vi "tvac_gui_chamber.vi"() -> ()   [LabVIEW 2016]
uses:
  <vilib>/httpClient/LabVIEWHTTPClient.lvlib
  <vilib>/httpClient/ClientHandle.ctl
  msg7171_linux.llb/send single message.vi
  <vilib>/httpClient/POSTBuffer.vi
panel:
  in  "read pressure":bool
  out "headers":string
  in  "ThermalProfile":bool
  in  "Read Zones":bool
  out "value":cluster{"ZoneSetPoint":dbl[], "ZoneTemp":dbl[]}
  in  "Read MCC":bool
  out "output cluster":T1
  out "Cluster":T2
  in  "Custom Graph Selector":i32
  in  "exit":bool
  in  "AlarmColor":u32(colorbox)
  in  "Alarm String":string
  in  "Plot Color":u32(colorbox)=16860
  in  "Temperature":dbl format="%#_13g"
  in  "TC Label":string
  in  "Graph ON/OFF":u32(colorbox)=4250624
  in  "index (col)":i32
  in  "index (row)":i32
  out "working array":bool[](array[boolean])
  in  "Local Debug":bool
  in  "Tab Control":enum32{"TCs", "Graphs", "Thermal Profile"}(tab)
  in  "Log/Linear Y-Axis":u16(ring) items=["Linear", "Log"]
  in  "Total Time":dbl
  in  "Set Time TC Graph":bool
  in  "Graphing Selection":u16(ring) items=["User Selection", "Graph All Thermocouples", "Clear Graph"]
  in  "Time Scale":u16(ring) items=["Minutes", "Hours", "Seconds"]
  out "Waveform Chart":waveform(dbl)[](graph)
  out "Thermocouples":T3(array[cluster])
  in  "Log/Linear Y-Axis 6":u16(ring) items=["Linear", "Log"]
  in  "Log/Linear Y-Axis 5":u16(ring) items=["Linear", "Log"]
  in  "Log/Linear Y-Axis 3":u16(ring) items=["Linear", "Log"]
  in  "Log/Linear Y-Axis 2":u16(ring) items=["Linear", "Log"]
  in  "Total Time 6":dbl
  in  "Set Time TC Graph 6":bool
  in  "Time Scale 6":u16(ring) items=["Minutes", "Hours", "Seconds"]
  in  "Total Time 5":dbl
  in  "Set Time TC Graph 5":bool
  in  "Time Scale 5":u16(ring) items=["Minutes", "Hours", "Seconds"]
  in  "Total Time 4":dbl
  in  "Set Time TC Graph 4":bool
  in  "Time Scale 4":u16(ring) items=["Minutes", "Hours", "Seconds"]
  in  "Total Time 3":dbl
  in  "Set Time TC Graph 3":bool
  in  "Time Scale 3":u16(ring) items=["Minutes", "Hours", "Seconds"]
  in  "Total Time 2":dbl
  in  "Set Time TC Graph 2":bool
  in  "Time Scale 2":u16(ring) items=["Minutes", "Hours", "Seconds"]
  in  "Log/Linear Y-Axis 1":u16(ring) items=["Linear", "Log"]
  in  "Total Time 1":dbl
  in  "Set Time TC Graph 1":bool
  in  "Time Scale 1":u16(ring) items=["Minutes", "Hours", "Seconds"]
  in  "Custom Chart 2 Selection":i32[](listbox)=[0]
  in  "Custom Chart 1 Selection":i32[](listbox)=[0]
  out "Custom Chart 1":waveform(dbl)[](graph)
  in  "Custom Chart 3 Selection":i32[](listbox)=[0]
  in  "Custom Chart 4 Selection":i32[](listbox)=[0]
  in  "Custom Chart 5 Selection":i32[](listbox)=[0]
  in  "Custom Chart 6 Selection":i32[](listbox)=[0]
  out "Custom Chart 2":waveform(dbl)[](graph)
  out "Custom Chart 3":waveform(dbl)[](graph)
  out "Custom Chart 4":waveform(dbl)[](graph)
  out "Custom Chart 5":waveform(dbl)[](graph)
  out "Custom Chart 6":waveform(dbl)[](graph)
  in  "Log/Linear Y-Axis 4":u16(ring) items=["Linear", "Log"]
  in  "Run Profile 2":bool
  in  "Run Profile":bool
  in  "Resume Profile":bool
  in  "Stop Profile":bool
  in  "Pause Profile":bool
  in  "Hold Profile":bool
  in  "Set Z 1":bool
  in  "Z3 Thermal Profile":i32(listbox)
  in  "Z2 Thermal Profile":i32(listbox)
  in  "Z1 Thermal Profile":i32(listbox)
  in  "Zone 3 Temp":u16(ring) items=["Average", "Minimum", "Maximum"]
  in  "Zone 2 Temp":u16(ring) items=["Average", "Minimum", "Maximum"]
  in  "Zone 1 Temp":u16(ring) items=["Average", "Minimum", "Maximum"]
  in  "Zone 1 TC":i32[](listbox)=[0]
  in  "Zone 2 TC":i32[](listbox)=[0]
  in  "Zone 3 TC":i32[](listbox)=[0]
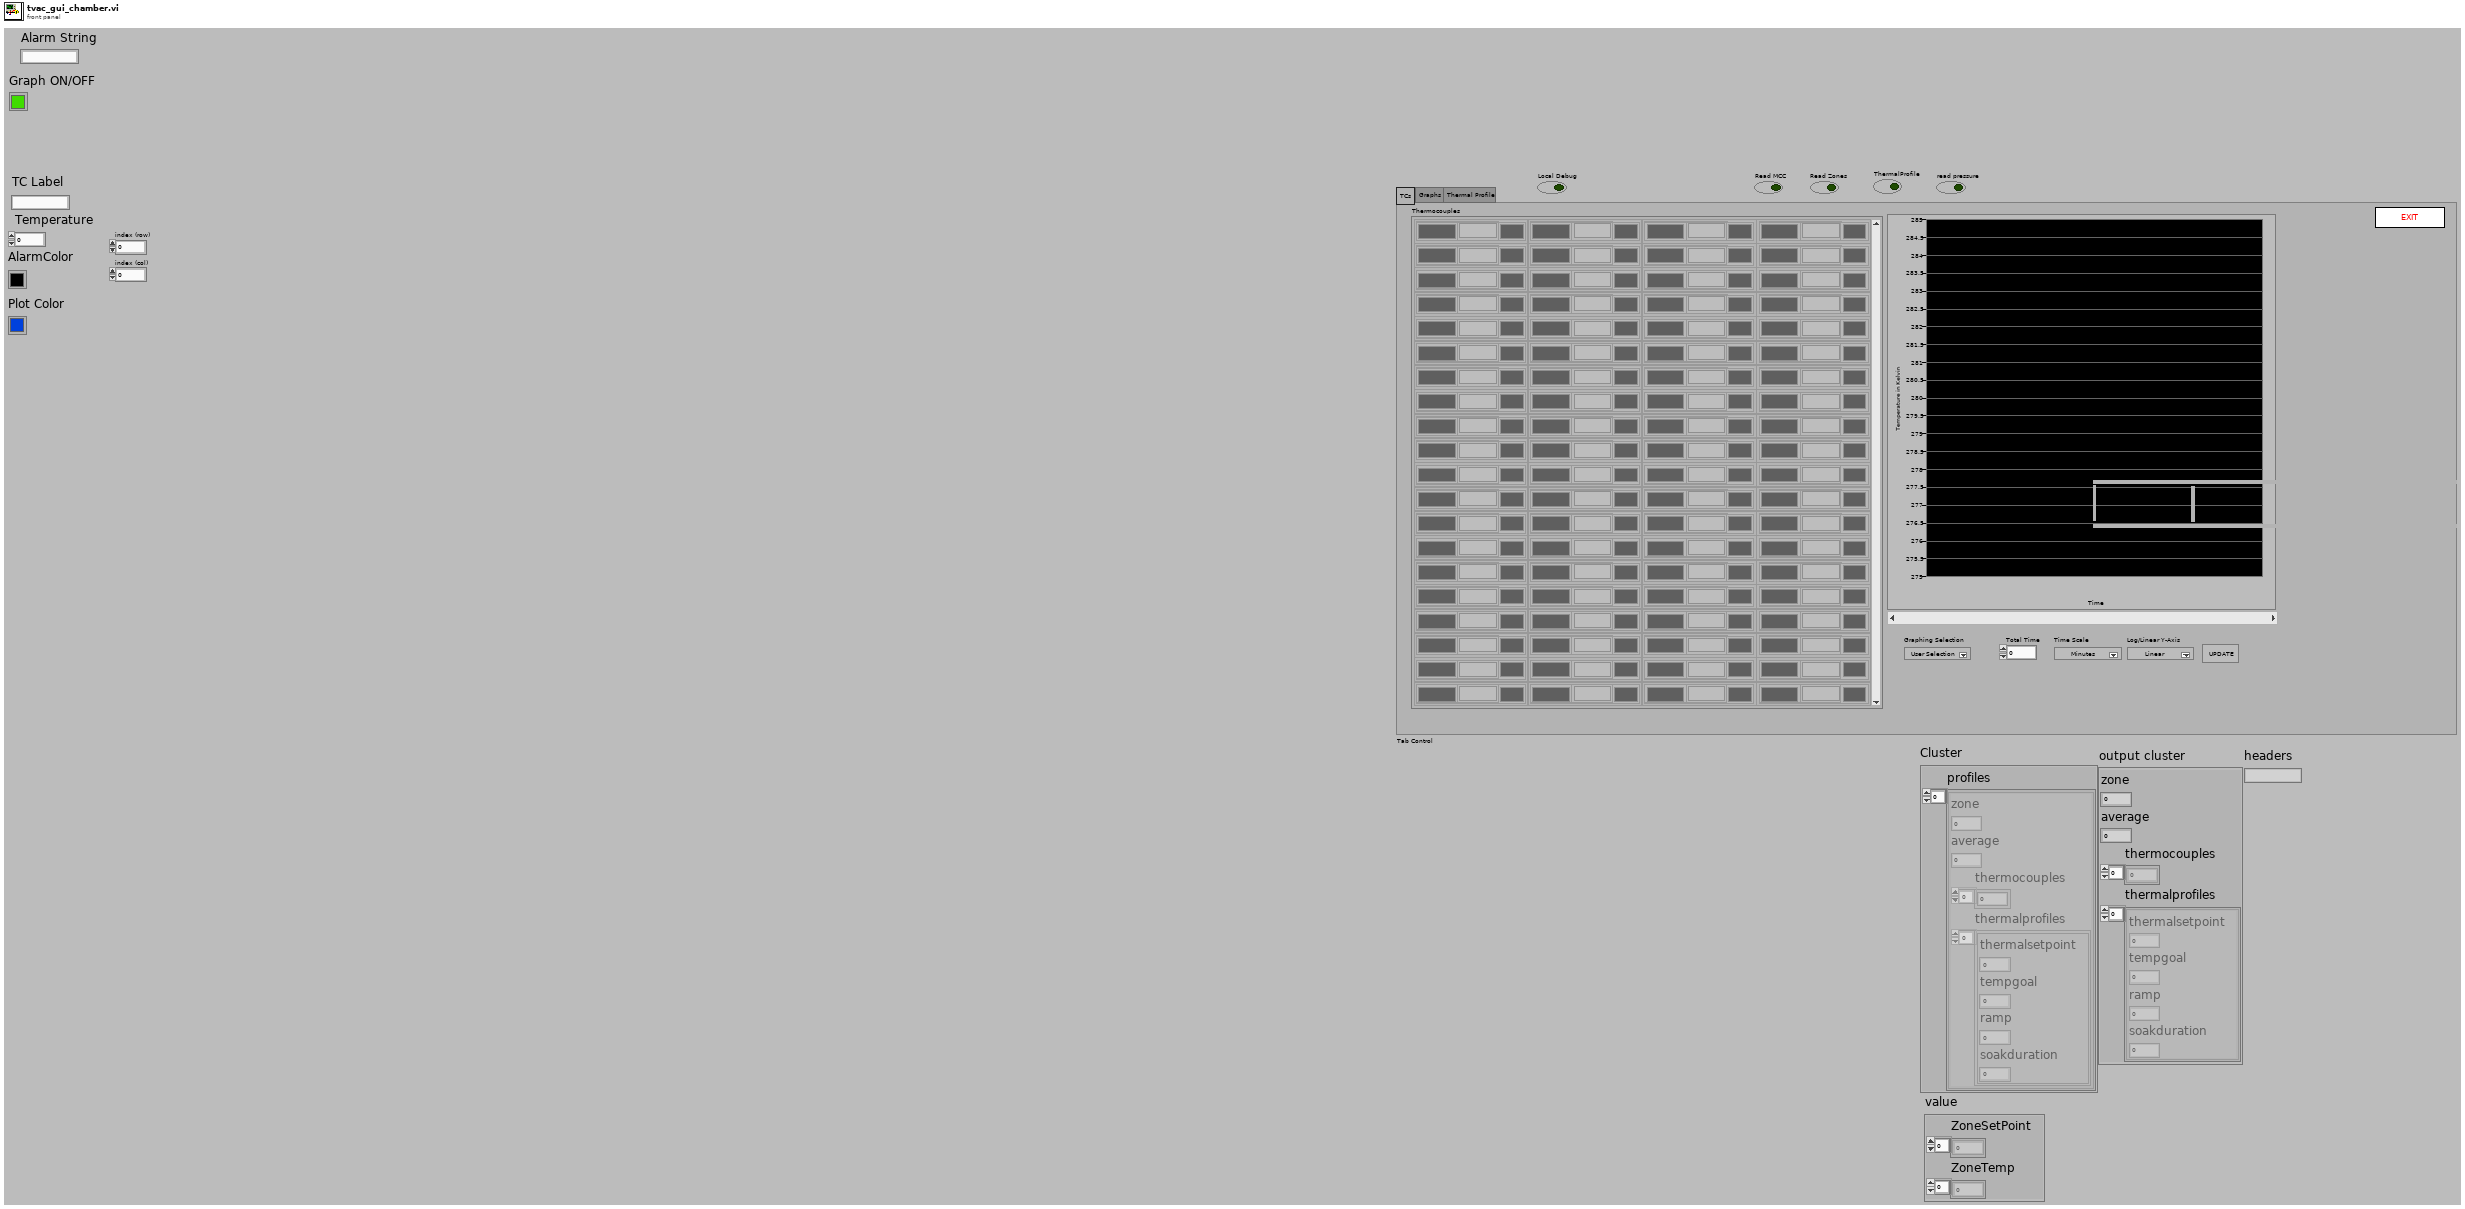
[diagram p1: front panel]
types:
  T1 = cluster{"zone":i32, "average":i32, "thermocouples":dbl[], "thermalprofiles":cluster{"thermalsetpoint":i32, "tempgoal":i32, "ramp":i32, "soakduration":i32}[]}
  T2 = cluster{"profiles":cluster{"zone":i32, "average":i32, "thermocouples":dbl[], "thermalprofiles":cluster{"thermalsetpoint":i32, "tempgoal":i32, "ramp":i32, "soakduration":i32}[]}[]}
  T3 = cluster{"TC Label":string, "Alarm Status":string, "Alarm Color":u32, "Temperature":string, "PlotColor":u32, "Graph On/Off":u32}[][]
  T4 = cluster{"Cp Stage 1 Temp":dbl[], "Cp Stage 2 Temp":dbl[], "Compressor Temp":dbl[]}
  T5 = typedef "LabVIEWHTTPClient.lvlib/ClientHandle.ctl" = refnum<k1>
  T6 = cluster{"go":bool, "Http session":T5, "URL prefex":string, "index (row)":i32, "index (col)":i32, "Graph ON/OFF":u32, "TC Label":string, "Temperature":dbl, "AlarmColor":u32, "Plot Color":u32, "Alarm String":string, "Thermocouples":cluster{"TC Label":string, "Alarm Status":string, "Alarm Color":u32, "Temperature":string, "PlotColor":u32, "Graph On/Off":u32}[][], "working array":bool[], "i":i32, "NumberTCs":i32, "Waveform Chart":waveform(dbl)[], "Custom Chart 1":waveform(dbl)[], "Pressure":dbl[], "numSensors":i32, "Database":dbl[], "PumpTemps":cluster{"Cp Stage 1 Temp":dbl[], "Cp Stage 2 Temp":dbl[], "Compressor Temp":dbl[]}, "Zones":dbl[], "Time":i32}
  T7 = cluster{"TC Label":string, "Alarm Status":string, "Alarm Color":u32, "Temperature":string, "PlotColor":u32, "Graph On/Off":u32}
  T8 = cluster{"CryoPressure":dbl, "ChamberPressure":dbl, "RoughingPressure":dbl}
  T9 = cluster{"DutyCycle":i32, "Stage1Temp":i32, "CryoPumpReadyState":cluster{"MotorOn":bool, "Ready":bool}, "PurgeValveState":bool, "RegenError":string, "RegenStep":string, "RoughingValveState":bool, "RoughingInterlock":cluster{"RoughingPermission":bool, "RoughingNeeded":bool, "Cryopumprunning":bool}, "Stage2Temp":i32, "Status":cluster{"PumpOn":bool, "RoughOpen":bool, "PurgeOpen":bool, "ThermocoupleGaugeOn":bool, "PowerFailureOccurred":bool}, "TcPressure":i32}
  T10 = cluster{"time":string, "TCs":cluster{"thermocouple":i32, "time":dbl, "temp":dbl, "working":bool, "alarm":i32}[]}
  T11 = cluster{"thermocouple":i32, "time":dbl, "temp":dbl, "working":bool, "alarm":i32}[]
  T12 = typedef "LVPositionTypeDef.ctl" = cluster{"Left":i32, "Top":i32}
  T13 = typedef "LVPoint32TypeDef.ctl" = cluster{"Horizontal":i32, "Vertical":i32}
  T14 = typedef "LVRangeTypeDef.ctl" = cluster{"Minimum":dbl, "Maximum":dbl, "Increment":dbl, "Minor Increment":dbl, "Start":dbl}
  T15 = cluster{"zone":i32, "average":i32, "thermocouples":dbl[], "thermalprofiles":cluster{"thermalsetpoint":i32, "tempgoal":i32, "ramp":i32, "soakduration":i32}[]}[]
  T16 = cluster{"profiles[0]":cluster{"zone":i32, "average":i32, "thermocouples":dbl[], "thermalprofiles":cluster{"thermalsetpoint":i32, "tempgoal":i32, "ramp":i32, "soakduration":i32}[]}, "profiles[1]":cluster{"zone":i32, "average":i32, "thermocouples":dbl[], "thermalprofiles":cluster{"thermalsetpoint":i32, "tempgoal":i32, "ramp":i32, "soakduration":i32}[]}, "profiles[2]":cluster{"zone":i32, "average":i32, "thermocouples":dbl[], "thermalprofiles":cluster{"thermalsetpoint":i32, "tempgoal":i32, "ramp":i32, "soakduration":i32}[]}, "profiles[3]":cluster{"zone":i32, "average":i32, "thermocouples":dbl[], "thermalprofiles":cluster{"thermalsetpoint":i32, "tempgoal":i32, "ramp":i32, "soakduration":i32}[]}, "profiles[4]":cluster{"zone":i32, "average":i32, "thermocouples":dbl[], "thermalprofiles":cluster{"thermalsetpoint":i32, "tempgoal":i32, "ramp":i32, "soakduration":i32}[]}, "profiles[5]":cluster{"zone":i32, "average":i32, "thermocouples":dbl[], "thermalprofiles":cluster{"thermalsetpoint":i32, "tempgoal":i32, "ramp":i32, "soakduration":i32}[]}, "profiles[6]":cluster{"zone":i32, "average":i32, "thermocouples":dbl[], "thermalprofiles":cluster{"thermalsetpoint":i32, "tempgoal":i32, "ramp":i32, "soakduration":i32}[]}, "profiles[7]":cluster{"zone":i32, "average":i32, "thermocouples":dbl[], "thermalprofiles":cluster{"thermalsetpoint":i32, "tempgoal":i32, "ramp":i32, "soakduration":i32}[]}, "profiles[8]":cluster{"zone":i32, "average":i32, "thermocouples":dbl[], "thermalprofiles":cluster{"thermalsetpoint":i32, "tempgoal":i32, "ramp":i32, "soakduration":i32}[]}}
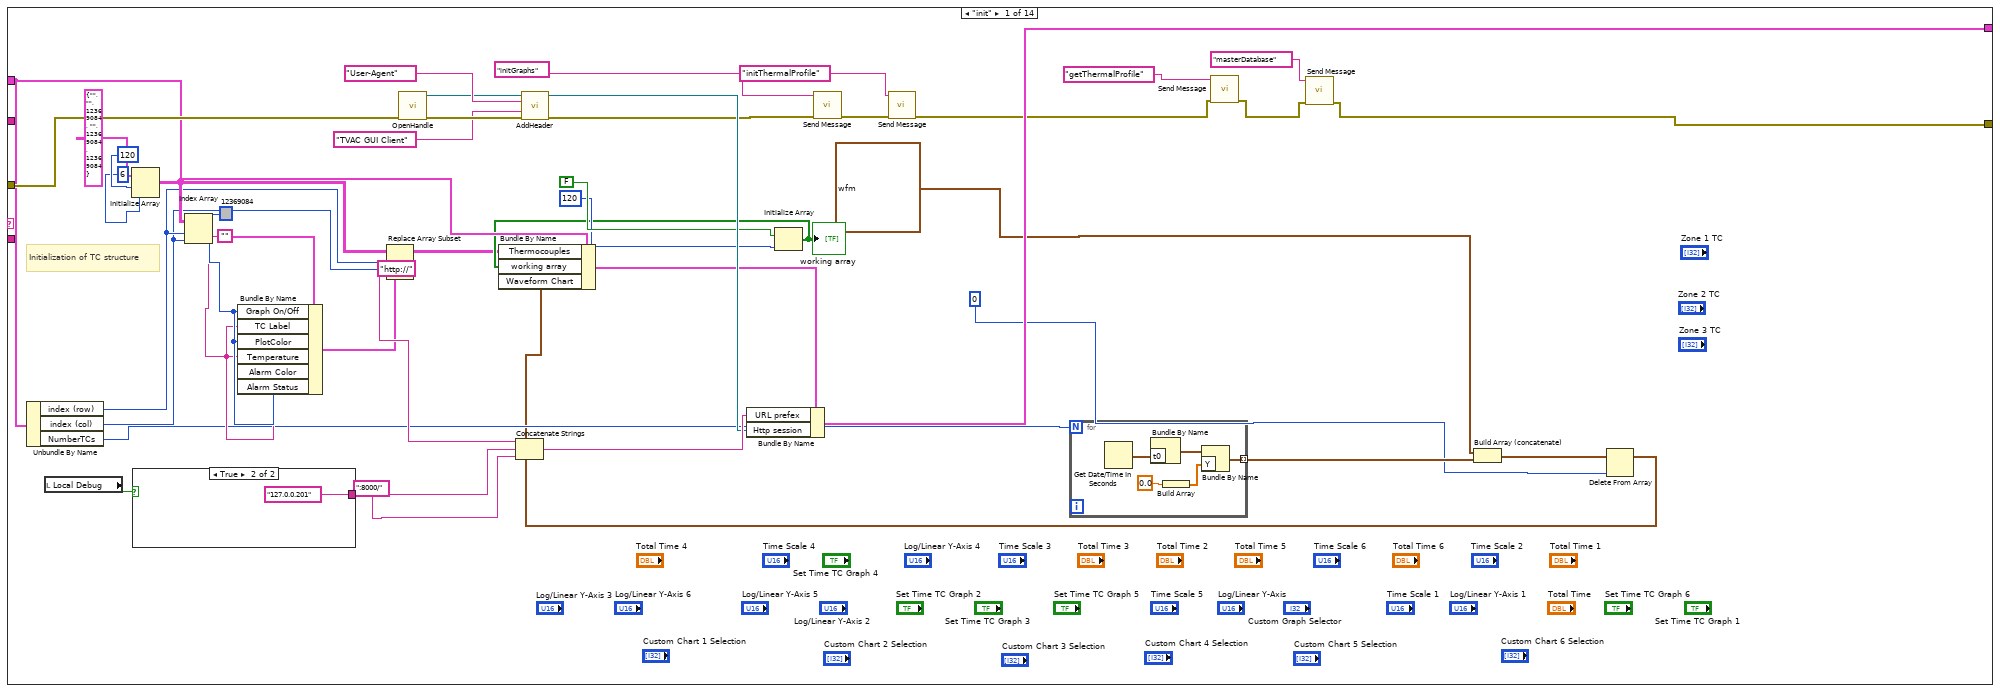
[diagram p2: hidden frame]
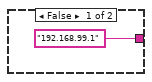
[diagram p3: hidden frame]
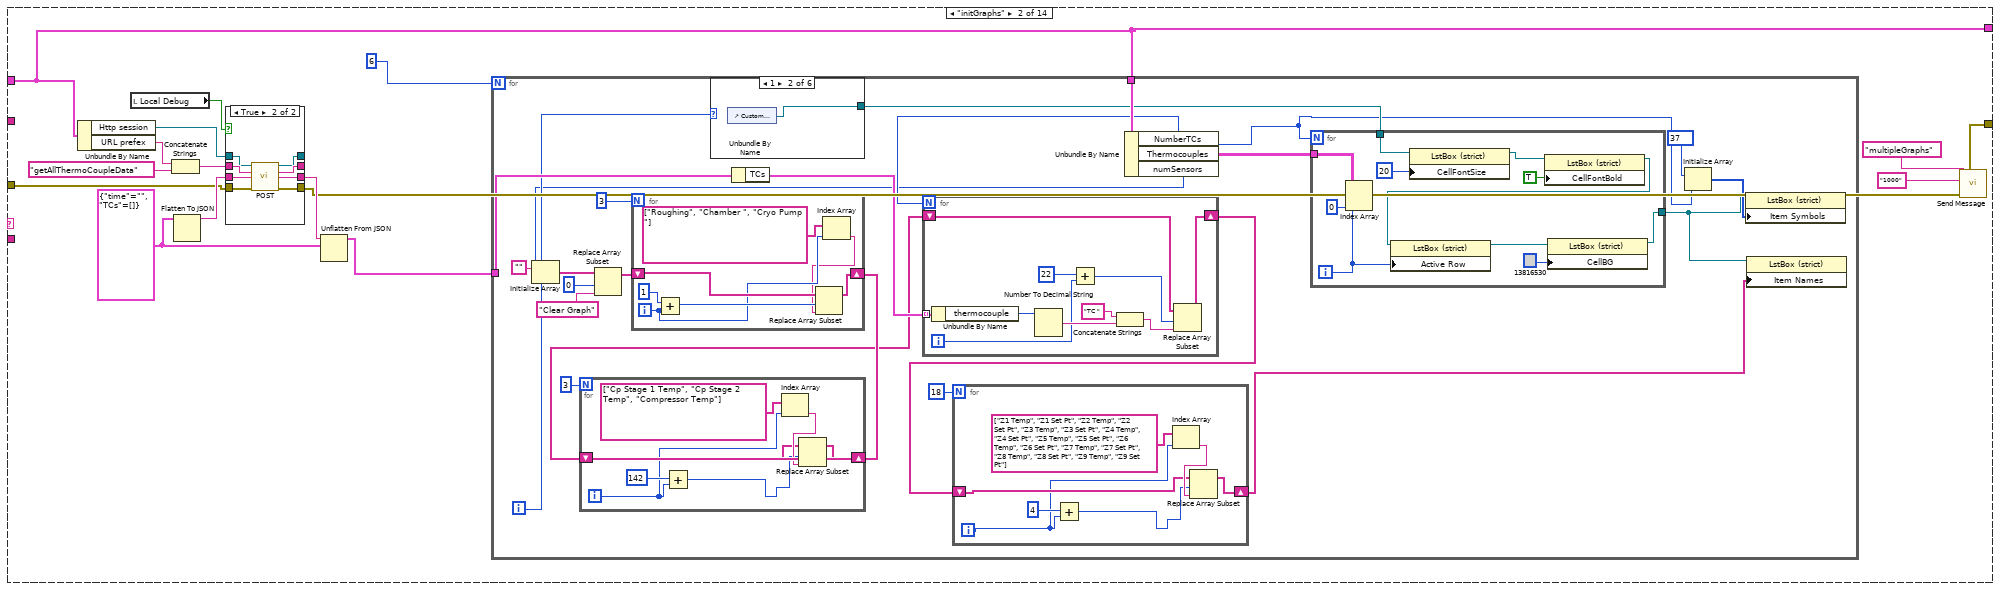
[diagram p4: hidden frame]
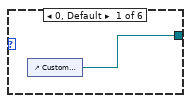
[diagram p5: hidden frame]
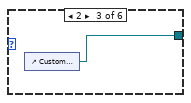
[diagram p6: hidden frame]
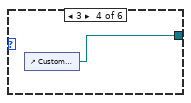
[diagram p7: hidden frame]
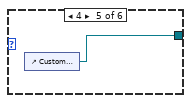
[diagram p8: hidden frame]
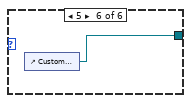
[diagram p9: hidden frame]
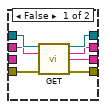
[diagram p10: hidden frame]
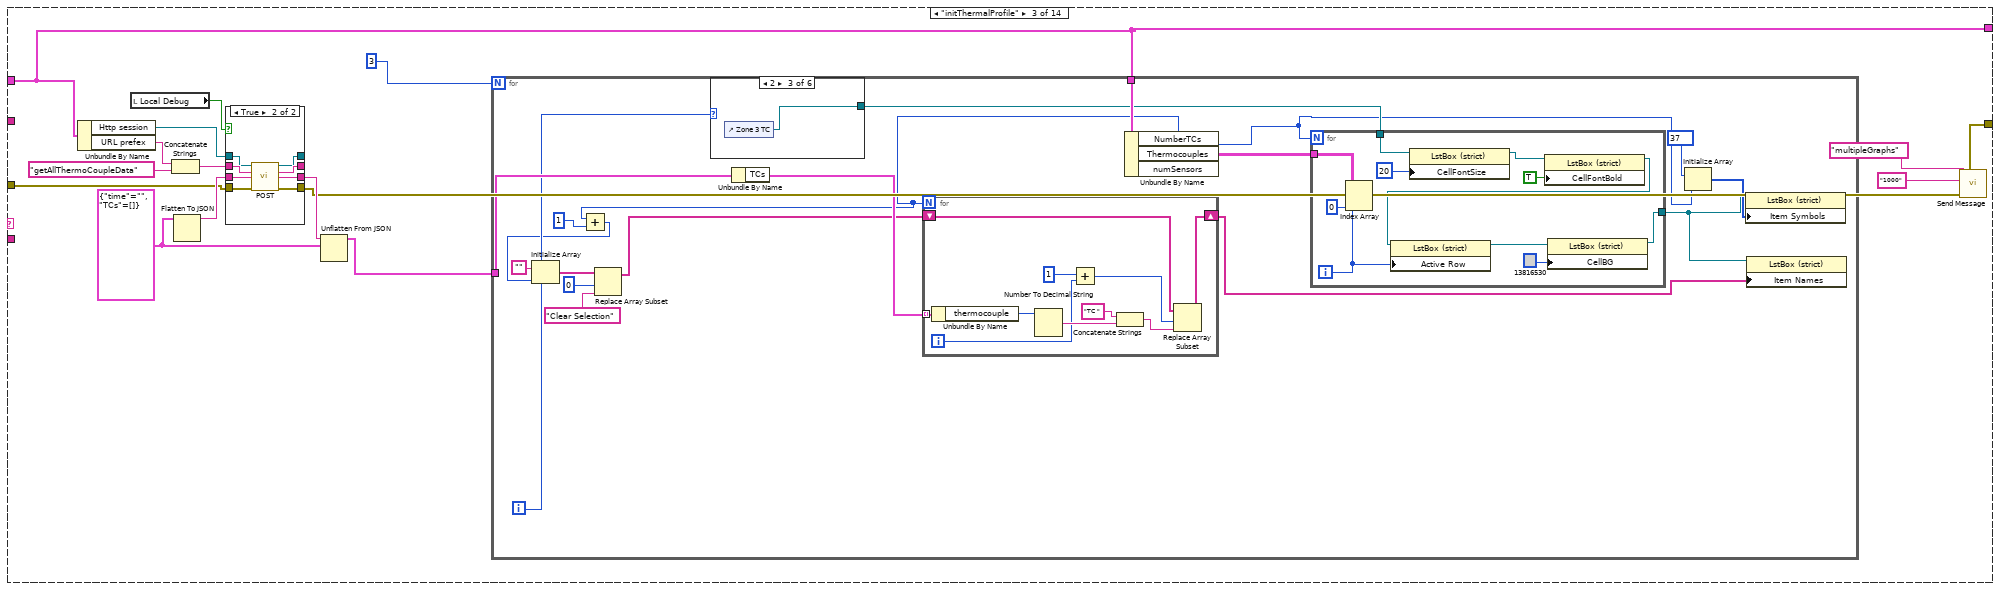
[diagram p11: hidden frame]
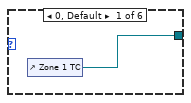
[diagram p12: hidden frame]
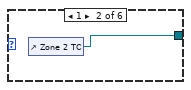
[diagram p13: hidden frame]
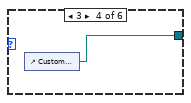
[diagram p14: hidden frame]
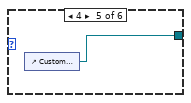
[diagram p15: hidden frame]
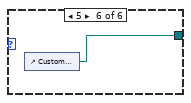
[diagram p16: hidden frame]
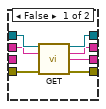
[diagram p17: hidden frame]
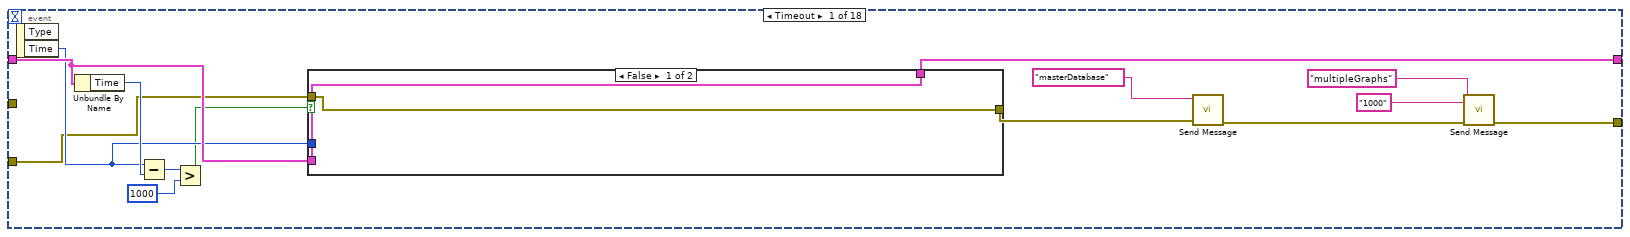
[diagram p18: hidden frame]
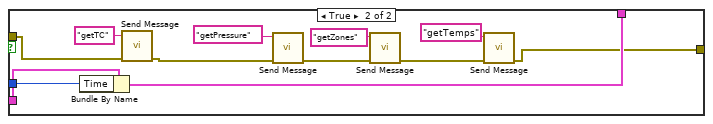
[diagram p19: hidden frame]
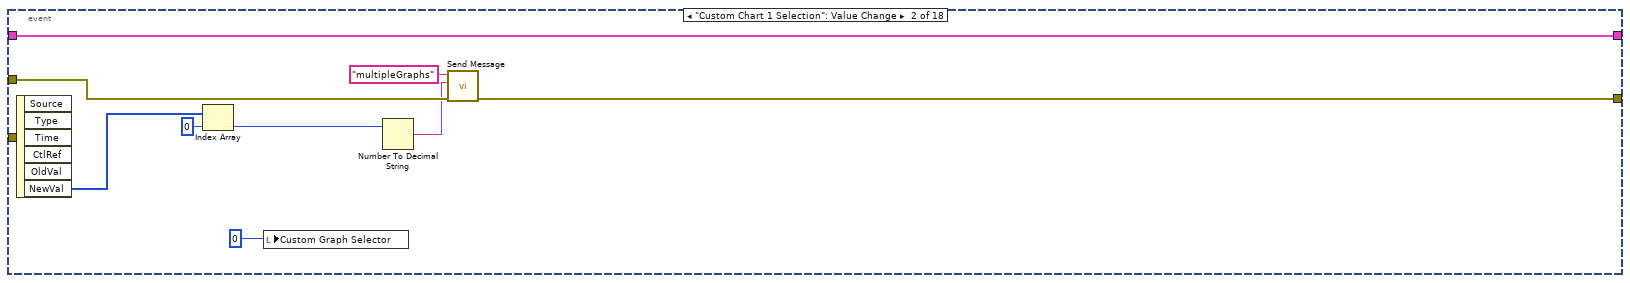
[diagram p20: hidden frame]
diagram:
  w3 = T4 {"Cp Stage 1 Temp"=[0.0], "Cp Stage 2 Temp"=[0.0], "Compressor Temp"=[0.0]}  # PumpTemps
  w6 = dbl[] [0.0, 0.0, 0.0]  # Pressure
  w26 = ""  # URL prefex
  w27 = T5 refnum  # Http session
  w28 = TRUE  # go
  n1 = call "Register Module.vi"() -> ("error out"=w24:errorcluster)  [unwired: 10 in, 1 out]
  n2 = call-poly "Send Message.vi"("error in (no error)"=w24, "event"="init") -> ("error out"=w23:errorcluster)  [unwired: 9 in]
  n3 = local read "Waveform Chart"() -> (w10:waveform(dbl)[])
  n4 = local read "Thermocouples"() -> (w8:T3)
  n5 = local read "Custom Chart 1"() -> (w7:waveform(dbl)[])
  n6 = Bundle("go"=w28, "Http session"=w27, "URL prefex"=w26, "index (row)"="index (row)", "index (col)"="index (col)", "Graph ON/OFF"="Graph ON/OFF", "TC Label"="TC Label", "Temperature"="Temperature", "AlarmColor"="AlarmColor", "Plot Color"="Plot Color", "Alarm String"="Alarm String", "Thermocouples"=w8, "working array"=bool[] [TRUE, TRUE, TRUE, TRUE, TRUE, TRUE, TRUE, TRUE, TRUE, TRUE, TRUE, TRUE, TRUE, TRUE, TRUE, TRUE, TRUE, TRUE, TRUE, TRUE, TRUE, TRUE, TRUE, TRUE, TRUE, TRUE, TRUE, TRUE, TRUE, TRUE, TRUE, TRUE, TRUE, TRUE, TRUE, TRUE, TRUE, TRUE, TRUE, TRUE, TRUE, TRUE, TRUE, TRUE, TRUE, TRUE, TRUE, TRUE, TRUE, TRUE, TRUE, TRUE, TRUE, TRUE, TRUE, TRUE, TRUE, TRUE, TRUE, TRUE, TRUE, TRUE, TRUE, TRUE, TRUE, TRUE, TRUE, TRUE, TRUE, TRUE, TRUE, TRUE, TRUE, TRUE, TRUE, TRUE, TRUE, TRUE, TRUE, TRUE, TRUE, TRUE, TRUE, TRUE, TRUE, TRUE, TRUE, TRUE, TRUE, TRUE, TRUE, TRUE, TRUE, TRUE, TRUE, TRUE, TRUE, TRUE, TRUE, TRUE, TRUE, TRUE, TRUE, TRUE, TRUE, TRUE, TRUE, TRUE, TRUE, TRUE, TRUE, TRUE, TRUE, TRUE, TRUE, TRUE, TRUE, TRUE, TRUE, TRUE], "i"=0, "NumberTCs"=120, "Waveform Chart"=w10, "Custom Chart 1"=w7, "Pressure"=w6, "numSensors"=145, "Database"=dbl[] [0.0, 1000.5841582194602, 1000.5841582194602, 1000.5841582194602, 0.6389895835935778, 0.7578061575842531, 1.153531014677555, 1.4572061556343079, 1.0192558642672256, 0.9245021790184325, 0.34311035179988925, 1.1970333160202968, 1.066989851322369, 0.5926593131154867, 0.7219240511326698, 1.0529790116491695, 1.4485694746891444, 0.9139060201605569, 0.7997359753068659, 0.6568795179977746, 0.8470104541419833, 1.0272585161866683, 0.6577301535824354, 0.645139941938139, 1.5235316442408067, 0.5128651184775285, 1.6421980587090137, 1.3961508335147417, 1.1242639015795428, 1.5954313466624428, 1.1919135255187876, 1.2615004458206727, 1.1320092264321664, 1.922759836270222, 1.1315561200367314, 1.4924621723754858, 0.6988771274186227, 1.069709701591943, 0.9920698240997152, 0.5395549253287656, 0.42891479657680576, 1.2794224940227927, 0.2687949632437338, 0.16127136772755854, 1.0174597006256374, 1.2079238230365172, 0.9745554383837218, 1.5348516925460962, 0.9488878852839246, 1.6634477658652282, 1.1924291951744272, 1.2231949298067308, 1.2223766746774598, 1.30664154589907, 1.2872878364107239, 0.5274250065177812, 0.7905999067114673, 1.2748974665085449, 1.216972941585413, 0.959115576325391, 0.5743502840762814, 0.8219540421676025, 0.613053899308251, 1.3785560870413707, 1.034117232127813, 1.1237698659753859, 1.4495548642149667, 0.6967905980938514, 0.6224497255665377, 1.6551326273040576, 1.2103048396824558, 0.6078721016951973, 1.3790669246280296, 0.5454332940871525, 1.5318777012492035, 1.2496539590411258, 0.9145395304446965, 1.3855381787793546, 1.0857600342029163, 1.3185833631438346, 0.9769688683142593, 1.026663691242448, 0.6744610422623843, 1.1965175398567691, 0.4847084945450119, 0.6435799980029115, 0.8079659363810663, 0.9130053929540112, 0.5271098423006861, 0.8088111736464799, 1.1455315536576556, 1.139809531926708, 1.5840192673434794, 1.0296748968089129, 1.7370669751200136, 1.3715484550405317, 0.3362063953932494, 1.0385868418202253, 1.4947740276021626, 1.0393600693910505, 0.8870410800672984, 1.2470388696569872, 0.9846724980375481, 0.9952471377109308, 1.0807485178906029, 1.1016630607035562, 1.3301039036808464, 0.8856852816151205, 0.4719509873120426, 0.5191430277856135, 0.12135113366044793, 0.4230478635224125, 1.1140562049976255, 1.5484968368781251, 1.1999891199114734, 1.8721302183420216, 1.071489235222563, 0.6260864330445979, 1.0305668002030492, 1.0223711899566386, 0.7842533472819472, 1.7301290335750898, 1.318694748426881, 0.6978662965493679], "PumpTemps"=w3, "Zones"=dbl[] [24.54828257301887, 25.0, 20.035959453954195, 26.0, 28.926820041278148, 27.0, 21.321976066931608, 28.0, 29.197600688359813, 29.0, 29.117373424110085, 30.0, 21.092914485312942, 31.0, 27.791581465649088, 32.0, 24.70861457288988, 33.0], "Time"=0) -> (w14:T6)  [unwired: 1 in]
  n7 = while {
    shift-left: w14 -> [w33]
    shift-right: [w30] -> _
    shift-right: [w31] -> w9
    shift-left: w23 -> [w38]
    stop <- w29 continue-if-true
    n8 = call "Get Message.vi"("error in (no error)"=w38) -> ("error out"=w36:errorcluster, "event buffer"=w37:string, "event"=w35:string, "source"=w34:string)  [unwired: 7 in]
    n9 = case shown="\"\", \"Idle\"" w35 {
      selector: w35 -> [_ _ _ _ _ _ _ _ _ _ _ _ _ w1431]
      tunnel: [w74 w95 w197 w279 w965 w1012 w1126 w1169 w1209 w1263 w1283 w1414 w1429 w1433] -> w30
      tunnel: w33 -> [w55 w95 w197 w280 w968 w1018 w1121 w1169 w1205 w1264 w1283 w1414 w1425 w1433]
      tunnel: w37 -> [_ _ _ _ _ _ _ _ _ _ w1284 _ _ _]
      tunnel: w36 -> [w77 w94 w196 w268 w967 w1034 w1120 w1167 w1210 w1269 _ _ w1428 w1432]
      tunnel: [w40 w90 w192 w278 w966 w1008 w1120 w1167 w1210 w1269 _ _ w1427 w1430] -> w32
      tunnel: w34 -> [_ _ _ _ _ _ _ _ _ _ _ _ _ _]
      frame "init" {
        w60 = ""
        w61 = u32 12369084 ("PlotColor")
        # "Initialization of TC structure"
        n10 = Unbundle By Name(w55) -> ("index (row)"=w63:i32, "index (col)"=w62:i32, "NumberTCs"=w52:i32)
        n11 = local read "Local Debug"() -> (w68:bool)
        n12 = Initialize Array(T7 {"TC Label"="", "Alarm Status"="", "Alarm Color"=12369084, "Temperature"="", "PlotColor"=12369084, "Graph On/Off"=12369084}, 120 ("dimension size"), 6 ("dimension size")) -> (w64:T3)
        n13 = case shown="True" w68 {
          tunnel: ["192.168.99.1" ("Address") "127.0.0.201" ("Address")] -> w69
          frame False {
          }
          frame True {
          }
        }
        n14 = Index Array(array=w64, index (row)=w63, index (col)=w62) -> (element=w59:T7)
        n15 = Bundle By Name(cluster=w59, "Graph On/Off"=w61, "TC Label"=w60, "PlotColor"=w61, "Temperature"=w60, "Alarm Color"=w61, "Alarm Status"=w60) -> (w58:T7)
        n16 = Replace Array Subset(array=w64, new element=w58, index (row)=w63, index (col)=w62) -> (w46:T3)
        n17 = call <vilib>:"OpenHandle.vi"("error in (no error)"=w77) -> ("client handle out"=w78:T5, "error out"=w81:errorcluster)  [unwired: 13 in]
        n18 = Concatenate Strings("http://" ("url"), w69, ":8000/" ("url")) -> (w73:string)
        n19 = call <vilib>:"AddHeader.vi"("client handle"=w78, "header"="User-Agent", "value"="TVAC GUI Client", "error in (no error)"=w81) -> ("client handle out"=w72:T5, "error out"=w71:errorcluster)  [unwired: 10 in]
        n20 = Initialize Array(FALSE ("Boolean"), 120 ("dimension size")) -> (w53:bool[])
        "working array" <- w53
        n21 = call-poly "Send Message.vi"("error in (no error)"=w71, "event"="initGraphs") -> ("error out"=w45:errorcluster)  [unwired: 9 in]
        n22 = call-poly "Send Message.vi"("error in (no error)"=w45, "event"="initThermalProfile") -> ("error out"=w43:errorcluster)  [unwired: 9 in]
        n23 = for {
          N: w52 -> [_]
          tunnel: [w82] -> w50 mode=indexing
          n24 = Get Date/Time In Seconds() -> (seconds since 1Jan1904=w86:timestamp)
          n25 = Bundle By Name("t0"=w86) -> (w83:waveform(dbl))  [unwired: 1 in]
          n26 = Build Array(0.0) -> (w85:dbl[])
          n27 = Bundle By Name(cluster=w83, "Y"=w85) -> (w82:waveform(dbl))
        }
        n28 = call-poly "Send Message.vi"("error in (no error)"=w43, "event"="getThermalProfile") -> ("error out"=w41:errorcluster)  [unwired: 9 in]
        n29 = call-poly "Send Message.vi"("error in (no error)"=w41, "event"="masterDatabase") -> ("error out"=w40:errorcluster)  [unwired: 9 in]
        n30 = Build Array (concatenate)(waveform(dbl) {"t0"=timestamp(0 s since 1904-01-01), "dt"=1.0, "Y"=[0.0]} ("element"), w50) -> (w51:waveform(dbl)[])
        n31 = Delete From Array(array=w51, index=0) -> (array with subset deleted=w49:waveform(dbl)[])  [unwired: 1 in, 1 out]
        n32 = Bundle By Name(cluster=w55, "Thermocouples"=w46, "working array"=w53, "Waveform Chart"=w49) -> (w54:T6)
        n33 = Bundle By Name(cluster=w54, "URL prefex"=w73, "Http session"=w72) -> (w74:T6)
      }
      frame "initGraphs" {
        w98 = T10 {"time"="", "TCs"=[]} ("Cluster")
        n34 = Unbundle By Name(w95) -> ("Http session"=w104:T5, "URL prefex"=w102:string)
        n35 = local read "Local Debug"() -> (w96:bool)
        n36 = Concatenate Strings(w102, "getAllThermoCoupleData" ("url")) -> (w103:string)
        n37 = Flatten To JSON(anything=w98) -> (JSON string=w97:string)  [unwired: 2 in, 1 out]
        n38 = case shown="True" w96 {
          tunnel: w94 -> [w182 w183]
          tunnel: [w181 w184] -> w91
          tunnel: [w180 w185] -> _
          tunnel: w104 -> [w179 w188]
          tunnel: w103 -> [w178 w189]
          tunnel: [w177 w186] -> w100
          tunnel: [w176 w187] -> _
          tunnel: w97 -> [_ w190]
          frame False {
            n39 = call <vilib>:"GET.vi"("client handle"=w179, "url"=w178, "error in (no error)"=w182) -> ("client handle out"=w180:T5, "headers"=w176:string, "body"=w177:string, "error out"=w181:errorcluster)  [unwired: 9 in]
          }
          frame True {
            n40 = call-poly <vilib>:"POST.vi"("client handle"=w188, "url"=w189, "buffer"=w190, "error in (no error)"=w183) -> ("client handle out"=w185:T5, "headers"=w187:string, "body"=w186:string, "error out"=w184:errorcluster)  [unwired: 8 in]
          }
        }
        n41 = Unflatten From JSON(JSON string=w100, type and defaults=w98) -> (value=w99:T10)  [unwired: 5 in, 1 out]
        n42 = for {
          N: 6 ("Numeric") -> [_]
          tunnel: w99 -> [w126]
          tunnel: w95 -> [w125]
          i -> [w108]
          n43 = case shown="1" w108 {
            tunnel: [w128 w129 w130 w131 w132 w133] -> w109
            frame 0, Default {
              n44 = control-ref of="Custom Chart 1 Selection"() -> (w128:refnum<vi>)
            }
            frame 1 {
              n45 = control-ref of="Custom Chart 2 Selection"() -> (w129:refnum<vi>)
            }
            frame 2 {
              n46 = control-ref of="Custom Chart 3 Selection"() -> (w130:refnum<vi>)
            }
            frame 3 {
              n47 = control-ref of="Custom Chart 4 Selection"() -> (w131:refnum<vi>)
            }
            frame 4 {
              n48 = control-ref of="Custom Chart 5 Selection"() -> (w132:refnum<vi>)
            }
            frame 5 {
              n49 = control-ref of="Custom Chart 6 Selection"() -> (w133:refnum<vi>)
            }
          }
          n50 = Unbundle By Name(w126) -> ("TCs"=w122:T11)
          n51 = Unbundle By Name(w125) -> ("NumberTCs"=w120:i32, "Thermocouples"=w127:T3, "numSensors"=w106:i32)
          n52 = Initialize Array("", w106) -> (w118:string[])
          n53 = Replace Array Subset(array=w118, new element="Clear Graph" ("new element/subarray"), index=0) -> (w115:string[])
          n54 = for {
            N: 3 -> [_]
            shift-right: [w153] -> w113
            shift-left: w115 -> [w154]
            i -> [w149]
            n55 = Add(x=1 ("index"), y=w149) -> (x+y=w151:i32)
            n56 = Index Array(array=string[] ["Roughing", "Chamber ", "Cryo Pump "], index=w149) -> (element=w148:string)
            n57 = Replace Array Subset(array=w154, new element=w148, index=w151) -> (w153:string[])
          }
          n58 = for {
            N: 3 -> [_]
            shift-right: [w144] -> w112
            shift-left: w113 -> [w145]
            i -> [w141]
            n59 = Add(x=142 ("index"), y=w141) -> (x+y=w142:i32)
            n60 = Index Array(array=string[] ["Cp Stage 1 Temp", "Cp Stage 2 Temp", "Compressor Temp"], index=w141) -> (element=w146:string)
            n61 = Replace Array Subset(array=w145, new element=w146, index=w142) -> (w144:string[])
          }
          n62 = for {
            N: w120 -> [_]
            tunnel: w122 -> [w161] mode=indexing
            shift-right: [w155] -> w105
            shift-left: w112 -> [w157]
            i -> [w159]
            n63 = Unbundle By Name(w161) -> ("thermocouple"=w162:i32)
            n64 = Number To Decimal String(number=w162) -> (decimal integer string=w164:string)  [unwired: 1 in]
            n65 = Add(x=22 ("index"), y=w159) -> (x+y=w158:i32)
            n66 = Concatenate Strings("TC " ("string"), w164) -> (w156:string)
            n67 = Replace Array Subset(array=w157, new element=w156, index=w158) -> (w155:string[])
          }
          n68 = for {
            N: 18 -> [_]
            shift-right: [w134] -> w111
            shift-left: w105 -> [w136]
            i -> [w135]
            n69 = Add(x=4 ("index"), y=w135) -> (x+y=w137:i32)
            n70 = Index Array(array=string[] ["Z1 Temp", "Z1 Set Pt", "Z2 Temp", "Z2 Set Pt", "Z3 Temp", "Z3 Set Pt", "Z4 Temp", "Z4 Set Pt", "Z5 Temp", "Z5 Set Pt", "Z6 Temp", "Z6 Set Pt", "Z7 Temp", "Z7 Set Pt", "Z8 Temp", "Z8 Set Pt", "Z9 Temp", "Z9 Set Pt"], index=w135) -> (element=w139:string)
            n71 = Replace Array Subset(array=w136, new element=w139, index=w137) -> (w134:string[])
          }
          n72 = for {
            N: w106 -> [_]
            tunnel: w127 -> [w175]
            tunnel: w109 -> [w169]
            tunnel: [w165] -> w107
            i -> [w172]
            n73 = Index Array(array=w175, index (row)=w172, index (col)=0 ("disabled index (col)")) -> ()  [unwired: 1 out]
            n74 = property on="Property Node" class="LstBox (strict)"(reference=w169, "CellFontSize"=u32 20 ("Active Row:Cell Font:Size")) -> (reference out=w168:refnum<vi>)  [unwired: 1 in, 1 out]
            n75 = property on="Property Node" class="LstBox (strict)"(reference=w168, "CellFontBold"=TRUE ("Active Row:Cell Font:Bold")) -> (reference out=w167:refnum<vi>)  [unwired: 1 in, 1 out]
            n76 = property on="Property Node" class="LstBox (strict)"(reference=w167, "Active Row"=w172) -> (reference out=w166:refnum<vi>)  [unwired: 1 in, 1 out]
            n77 = property on="Property Node" class="LstBox (strict)"(reference=w166, "CellBG"=u32 13816530 ("Active Row:Cell Background Color")) -> (reference out=w165:refnum<vi>)  [unwired: 1 in, 1 out]
          }
          n78 = Initialize Array(37, w106) -> (w123:i32[])
          n79 = property on="Property Node" class="LstBox (strict)"(reference=w107, "Item Symbols"=w123) -> ()  [unwired: 1 in, 2 out]
          n80 = property on="Property Node" class="LstBox (strict)"(reference=w107, "Item Names"=w111) -> ()  [unwired: 1 in, 2 out]
        }
        n81 = call-poly "Send Message.vi"("error in (no error)"=w91, "event buffer"="1000", "event"="multipleGraphs") -> ("error out"=w90:errorcluster)  [unwired: 8 in]
      }
      frame "initThermalProfile" {
        w200 = T10 {"time"="", "TCs"=[]} ("Cluster")
        n82 = Unbundle By Name(w197) -> ("Http session"=w206:T5, "URL prefex"=w204:string)
        n83 = local read "Local Debug"() -> (w198:bool)
        n84 = Concatenate Strings(w204, "getAllThermoCoupleData" ("url")) -> (w205:string)
        n85 = Flatten To JSON(anything=w200) -> (JSON string=w199:string)  [unwired: 2 in, 1 out]
        n86 = case shown="True" w198 {
          tunnel: w196 -> [w259 w260]
          tunnel: [w258 w261] -> w193
          tunnel: [w257 w262] -> _
          tunnel: w206 -> [w256 w265]
          tunnel: w205 -> [w255 w266]
          tunnel: [w254 w263] -> w202
          tunnel: [w253 w264] -> _
          tunnel: w199 -> [_ w267]
          frame False {
            n87 = call <vilib>:"GET.vi"("client handle"=w256, "url"=w255, "error in (no error)"=w259) -> ("client handle out"=w257:T5, "headers"=w253:string, "body"=w254:string, "error out"=w258:errorcluster)  [unwired: 9 in]
          }
          frame True {
            n88 = call-poly <vilib>:"POST.vi"("client handle"=w265, "url"=w266, "buffer"=w267, "error in (no error)"=w260) -> ("client handle out"=w262:T5, "headers"=w264:string, "body"=w263:string, "error out"=w261:errorcluster)  [unwired: 8 in]
          }
        }
        n89 = Unflatten From JSON(JSON string=w202, type and defaults=w200) -> (value=w201:T10)  [unwired: 5 in, 1 out]
        n90 = for {
          N: 3 ("Numeric") -> [_]
          tunnel: w201 -> [w224]
          tunnel: w197 -> [w223]
          i -> [w214]
          n91 = case shown="2" w214 {
            tunnel: [w226 w227 w228 w229 w230 w231] -> w215
            frame 0, Default {
              n92 = control-ref of="Zone 1 TC"() -> (w226:refnum<vi>)
            }
            frame 1 {
              n93 = control-ref of="Zone 2 TC"() -> (w227:refnum<vi>)
            }
            frame 2 {
              n94 = control-ref of="Zone 3 TC"() -> (w228:refnum<vi>)
            }
            frame 3 {
              n95 = control-ref of="Custom Chart 4 Selection"() -> (w229:refnum<vi>)
            }
            frame 4 {
              n96 = control-ref of="Custom Chart 5 Selection"() -> (w230:refnum<vi>)
            }
            frame 5 {
              n97 = control-ref of="Custom Chart 6 Selection"() -> (w231:refnum<vi>)
            }
          }
          n98 = Unbundle By Name(w224) -> ("TCs"=w220:T11)
          n99 = Unbundle By Name(w223) -> ("NumberTCs"=w209:i32, "Thermocouples"=w225:T3, "numSensors"=w212:i32)
          n100 = Add(x=w209, y=1 ("index")) -> (x+y=w207:i32)
          n101 = Initialize Array("", w207) -> (w218:string[])
          n102 = Replace Array Subset(array=w218, new element="Clear Selection" ("new element/subarray"), index=0) -> (w211:string[])
          n103 = for {
            N: w209 -> [_]
            tunnel: w220 -> [w238] mode=indexing
            shift-right: [w232] -> w210
            shift-left: w211 -> [w234]
            i -> [w236]
            n104 = Unbundle By Name(w238) -> ("thermocouple"=w239:i32)
            n105 = Number To Decimal String(number=w239) -> (decimal integer string=w241:string)  [unwired: 1 in]
            n106 = Add(x=1 ("index"), y=w236) -> (x+y=w235:i32)
            n107 = Concatenate Strings("TC " ("string"), w241) -> (w233:string)
            n108 = Replace Array Subset(array=w234, new element=w233, index=w235) -> (w232:string[])
          }
          n109 = for {
            N: w212 -> [_]
            tunnel: w225 -> [w252]
            tunnel: w215 -> [w246]
            tunnel: [w242] -> w213
            i -> [w249]
            n110 = Index Array(array=w252, index (row)=w249, index (col)=0 ("disabled index (col)")) -> ()  [unwired: 1 out]
            n111 = property on="Property Node" class="LstBox (strict)"(reference=w246, "CellFontSize"=u32 20 ("Active Row:Cell Font:Size")) -> (reference out=w245:refnum<vi>)  [unwired: 1 in, 1 out]
            n112 = property on="Property Node" class="LstBox (strict)"(reference=w245, "CellFontBold"=TRUE ("Active Row:Cell Font:Bold")) -> (reference out=w244:refnum<vi>)  [unwired: 1 in, 1 out]
            n113 = property on="Property Node" class="LstBox (strict)"(reference=w244, "Active Row"=w249) -> (reference out=w243:refnum<vi>)  [unwired: 1 in, 1 out]
            n114 = property on="Property Node" class="LstBox (strict)"(reference=w243, "CellBG"=u32 13816530 ("Active Row:Cell Background Color")) -> (reference out=w242:refnum<vi>)  [unwired: 1 in, 1 out]
          }
          n115 = Initialize Array(37, w212) -> (w221:i32[])
          n116 = property on="Property Node" class="LstBox (strict)"(reference=w213, "Item Symbols"=w221) -> ()  [unwired: 1 in, 2 out]
          n117 = property on="Property Node" class="LstBox (strict)"(reference=w213, "Item Names"=w210) -> ()  [unwired: 1 in, 2 out]
        }
        n118 = call-poly "Send Message.vi"("error in (no error)"=w193, "event buffer"="1000", "event"="multipleGraphs") -> ("error out"=w192:errorcluster)  [unwired: 8 in]
      }
      frame "", "Idle" {
        n119 = control-ref of="Thermocouples"() -> (w277:refnum<vi>)
        n120 = property on="Property Node" class="Arr (strict)"(reference=w277) -> ("Position"=w276:T12)  [unwired: 1 in, 2 out]
        n121 = Unbundle By Name(w276) -> ("Left"=w275:i32, "Top"=w273:i32)
        n122 = Add(x=4, y=w275) -> (x+y=w271:i32)
        n123 = Add(x=w273, y=23 ("x")) -> (x+y=w270:i32)
        n124 = event shown="[8] \"Thermocouples\": Mouse Down" {
          selector: _ -> [_ _ _ _ _ _ _ _ _ _ _ _ _ _ _ _ _ _]
          dyn-events: _ -> [_ _ _ _ _ _ _ _ _ _ _ _ _ _ _ _ _ _]
          timeout: 200 ("milliseconds to wait") -> [_ _ _ _ _ _ _ _ _ _ _ _ _ _ _ _ _ _]
          tunnel: w268 -> [_ w314 w323 w332 w341 w350 w359 w364 w379 w472 w536 w597 w658 w719 w780 w841 w902 w961]
          tunnel: [w294 w313 w322 w331 w340 w349 w358 w363 w379 w472 w536 w597 w658 w719 w780 w841 w902 w959] -> w278
          tunnel: [w287 w315 w324 w333 w342 w351 w360 w368 w380 w466 w537 w598 w659 w720 w781 w842 w903 w962] -> w279
          tunnel: w280 -> [w288 w315 w324 w333 w342 w351 w360 w368 w381 w468 w537 w598 w659 w720 w781 w842 w903 w962]
          tunnel: w271 -> [_ _ _ _ _ _ _ _ w378 _ _ _ _ _ _ _ _ _]
          tunnel: w270 -> [_ _ _ _ _ _ _ _ w375 _ _ _ _ _ _ _ _ _]
          tunnel: w268 -> [w282 _ _ _ _ _ _ _ _ _ _ _ _ _ _ _ _ _]
          event Timeout {
            n125 = event-data() -> ("Time"=w286:u32)  [unwired: 1 in, 1 out]
            n126 = Unbundle By Name(w288) -> ("Time"=w291:i32)
            n127 = Subtract(x=w286, y=w291) -> (x-y=w290:u32)
            n128 = Greater?(x=w290, y=u32 1000 ("millisecond multiple")) -> (0:w281:bool)
            n129 = case shown="False" w281 {
              tunnel: w288 -> [w296 w304]
              tunnel: [w296 w303] -> w287
              tunnel: w286 -> [_ w302]
              tunnel: [w295 w301] -> w285
              tunnel: w282 -> [w295 w299]
              frame False {
              }
              frame True {
                n130 = Bundle By Name(cluster=w304, "Time"=w302) -> (w303:T6)
                n131 = call-poly "Send Message.vi"("error in (no error)"=w299, "event"="getTC") -> ("error out"=w297:errorcluster)  [unwired: 9 in]
                n132 = call-poly "Send Message.vi"("error in (no error)"=w297, "event"="getPressure") -> ("error out"=w308:errorcluster)  [unwired: 9 in]
                n133 = call-poly "Send Message.vi"("error in (no error)"=w308, "event"="getZones") -> ("error out"=w306:errorcluster)  [unwired: 9 in]
                n134 = call-poly "Send Message.vi"("error in (no error)"=w306, "event"="getTemps") -> ("error out"=w301:errorcluster)  [unwired: 9 in]
              }
            }
            n135 = call-poly "Send Message.vi"("error in (no error)"=w285, "event"="masterDatabase") -> ("error out"=w284:errorcluster)  [unwired: 9 in]
            n136 = call-poly "Send Message.vi"("error in (no error)"=w284, "event buffer"="1000", "event"="multipleGraphs") -> ("error out"=w294:errorcluster)  [unwired: 8 in]
          }
          event "Custom Chart 1 Selection": Value Change {
            n137 = event-data() -> ("NewVal"=w316:i32[])  [unwired: 1 in, 5 out]
            n138 = Index Array(array=w316, index=0) -> (element=w310:i32)
            n139 = local write "Custom Graph Selector"(0) -> ()
            n140 = Number To Decimal String(number=w310) -> (decimal integer string=w311:string)  [unwired: 1 in]
            n141 = call-poly "Send Message.vi"("error in (no error)"=w314, "event buffer"=w311, "event"="multipleGraphs") -> ("error out"=w313:errorcluster)  [unwired: 8 in]
          }
          event "Custom Chart 2 Selection": Value Change {
            n142 = event-data() -> ("NewVal"=w325:i32[])  [unwired: 1 in, 5 out]
            n143 = Index Array(array=w325, index=0) -> (element=w319:i32)
            n144 = local write "Custom Graph Selector"(1) -> ()
            n145 = Number To Decimal String(number=w319) -> (decimal integer string=w320:string)  [unwired: 1 in]
            n146 = call-poly "Send Message.vi"("error in (no error)"=w323, "event buffer"=w320, "event"="multipleGraphs") -> ("error out"=w322:errorcluster)  [unwired: 8 in]
          }
          event "Custom Chart 3 Selection": Value Change {
            n147 = event-data() -> ("NewVal"=w334:i32[])  [unwired: 1 in, 5 out]
            n148 = Index Array(array=w334, index=0) -> (element=w328:i32)
            n149 = local write "Custom Graph Selector"(2) -> ()
            n150 = Number To Decimal String(number=w328) -> (decimal integer string=w329:string)  [unwired: 1 in]
            n151 = call-poly "Send Message.vi"("error in (no error)"=w332, "event buffer"=w329, "event"="multipleGraphs") -> ("error out"=w331:errorcluster)  [unwired: 8 in]
          }
          event "Custom Chart 4 Selection": Value Change {
            n152 = event-data() -> ("NewVal"=w343:i32[])  [unwired: 1 in, 5 out]
            n153 = Index Array(array=w343, index=0) -> (element=w337:i32)
            n154 = local write "Custom Graph Selector"(3) -> ()
            n155 = Number To Decimal String(number=w337) -> (decimal integer string=w338:string)  [unwired: 1 in]
            n156 = call-poly "Send Message.vi"("error in (no error)"=w341, "event buffer"=w338, "event"="multipleGraphs") -> ("error out"=w340:errorcluster)  [unwired: 8 in]
          }
          event "Custom Chart 5 Selection": Value Change {
            n157 = event-data() -> ("NewVal"=w352:i32[])  [unwired: 1 in, 5 out]
            n158 = Index Array(array=w352, index=0) -> (element=w346:i32)
            n159 = local write "Custom Graph Selector"(4) -> ()
            n160 = Number To Decimal String(number=w346) -> (decimal integer string=w347:string)  [unwired: 1 in]
            n161 = call-poly "Send Message.vi"("error in (no error)"=w350, "event buffer"=w347, "event"="multipleGraphs") -> ("error out"=w349:errorcluster)  [unwired: 8 in]
          }
          event "Custom Chart 6 Selection": Value Change {
            n162 = event-data() -> ("NewVal"=w361:i32[])  [unwired: 1 in, 5 out]
            n163 = Index Array(array=w361, index=0) -> (element=w355:i32)
            n164 = local write "Custom Graph Selector"(5) -> ()
            n165 = Number To Decimal String(number=w355) -> (decimal integer string=w356:string)  [unwired: 1 in]
            n166 = call-poly "Send Message.vi"("error in (no error)"=w359, "event buffer"=w356, "event"="multipleGraphs") -> ("error out"=w358:errorcluster)  [unwired: 8 in]
          }
          event "Tab Control": Value Change {
            n167 = event-data() -> ("NewVal"=w367:enum32{"TCs", "Graphs", "Thermal Profile"})  [unwired: 1 in, 5 out]
            n168 = Equal?(x=w367, y=enum16{"Graphs"}."Graphs") -> (x = y?=w365:bool)
            n169 = case shown="True" w365 {
              tunnel: w364 -> [w369 w371]
              tunnel: [w369 w370] -> w363
              frame False {
              }
              frame True {
                n170 = call-poly "Send Message.vi"("error in (no error)"=w371, "event"="getGraphs") -> ("error out"=w370:errorcluster)  [unwired: 9 in]
              }
            }
          }
          event "Thermocouples": Mouse Down {
            n171 = event-data() -> ("CtlRef"=w383:refnum<vi>, "Coords"=w388:T13)  [unwired: 1 in, 3 out]
            n172 = Unbundle By Name(w388) -> ("Horizontal"=w386:i32, "Vertical"=w385:i32)
            n173 = Add(x=783 ("y"), y=w378) -> (x+y=w373:i32)
            n174 = Less?(x=w386, y=w373) -> (x < y?=w387:bool)
            n175 = Add(x=w375, y=854) -> (x+y=w374:i32)
            n176 = Less?(x=w385, y=w374) -> (x < y?=w384:bool)
            n177 = And(x=w387, y=w384) -> (x .and. y?=w382:bool)
            n178 = case shown="True" w382 {
              tunnel: w383 -> [_ w430]
              tunnel: w381 -> [_ w402]
              tunnel: w381 -> [w389 w400]
              tunnel: [w389 w392] -> w380
              tunnel: w378 -> [_ w391]
              tunnel: w375 -> [_ w390]
              frame False {
              }
              frame True {
                w424 = u16 0 items=["User Selection", "Graph All Thermocouples", "Clear Graph"] ("Graphing Selection")
                n179 = property class="Arr (strict)"(reference=w430) -> ("Array Element.Position"=w422:T12)  [unwired: 1 in, 2 out]
                n180 = local write "Graphing Selection"(w424) -> ()
                n181 = Unbundle By Name(w422) -> ("Left"=w420:i32, "Top"=w423:i32)
                n182 = property on="Thermocouples" class="Arr (strict)"() -> ("Index Values"=w414:u32[])  [unwired: 2 in, 2 out]
                n183 = Subtract(x=w391, y=w420) -> (x-y=w419:i32)
                n184 = Subtract(x=w390, y=w423) -> (x-y=w411:i32)
                n185 = Absolute Value(x=w411) -> (abs(x)=w421:i32)
                n186 = Index Array(array=w414, index=0) -> (element=w410:u32)
                n187 = To Byte Integer(number=w410) -> (8bit integer=w409:i8)
                n188 = Absolute Value(x=w419) -> (abs(x)=w418:i32)
                n189 = local read "Thermocouples"() -> (w393:T3)
                n190 = Quotient & Remainder(x=w421, y=42) -> (floor(x/y)=w408:i32)  [unwired: 1 out]
                n191 = Add(x=w409, y=w408) -> (x+y=w395:i32)
                n192 = Quotient & Remainder(x=w418, y=197 ("Numeric 2")) -> (floor(x/y)=w394:i32)  [unwired: 1 out]
                n193 = Index Array(array=w393, index (row)=w395, index (col)=w394) -> (element=w396:T7)
                n194 = Multiply(x=4, y=w395) -> (x*y=w415:i32)
                n195 = Unbundle By Name(w402) -> ("working array"=w401:bool[])  [unwired: 1 out]
                n196 = Unbundle By Name(w396) -> ("Alarm Color"=w428:u32, "Graph On/Off"=w427:u32, "TC Label"=w426:string, "PlotColor"=w407:u32, "Alarm Status"=w425:string, "Temperature"=w398:string)
                n197 = Add(x=w415, y=w394) -> (x+y=w404:i32)
                n198 = control-ref of="Waveform Chart"() -> (w429:refnum<vi>)
                n199 = Index Array(array=w401, index=w404) -> (element=w403:bool)
                n200 = Decimal String To Number(string=w398) -> ()  [unwired: 2 in, 2 out]
                n201 = Equal?(x=w427, y=u32 12369084) -> (x = y?=w405:bool)
                n202 = case shown="True" w403 {
                  selector: w403 -> [_ w436]
                  tunnel: w429 -> [_ w442]
                  tunnel: w428 -> [_ w441]
                  tunnel: w426 -> [_ w440]
                  tunnel: w425 -> [_ w439]
                  tunnel: w404 -> [_ w432]
                  tunnel: w407 -> [_ w438]
                  tunnel: w405 -> [_ w437]
                  tunnel: w398 -> [_ w435]
                  tunnel: [w431 w434] -> w397
                  tunnel: w396 -> [w431 w433]
                  frame False {
                  }
                  frame True {
                    n203 = case shown="True" w437 {
                      tunnel: w442 -> [w452 w463]
                      tunnel: w441 -> [w446 w458]
                      tunnel: w440 -> [w447 w457]
                      tunnel: w439 -> [w448 w459]
                      tunnel: w438 -> [_ w461]
                      tunnel: w436 -> [_ _]
                      tunnel: w435 -> [w449 w460]
                      tunnel: [w444 w456] -> w434
                      tunnel: w433 -> [w445 w455]
                      tunnel: w432 -> [w443 w454]
                      frame False {
                        w450 = u32 12369084
                        n204 = property on="Property Node" class="WFChart (strict)"(reference=w452, "Active Plot"=w443) -> (reference out=w453:refnum<vi>)  [unwired: 1 in, 1 out]
                        n205 = Bundle By Name(cluster=w445, "Graph On/Off"=w450, "TC Label"=w447, "PlotColor"=w450, "Temperature"=w449, "Alarm Color"=w446, "Alarm Status"=w448) -> (w444:T7)
                        n206 = property class="WFChart (strict)"(reference=w453, "Plot.Visible?"=FALSE ("Plot.Visible")) -> ()  [unwired: 1 in, 2 out]
                      }
                      frame True {
                        n207 = property class="WFChart (strict)"(reference=w463, "Active Plot"=w454) -> (reference out=w464:refnum<vi>)  [unwired: 1 in, 1 out]
                        n208 = Bundle By Name(cluster=w455, "Graph On/Off"=u32 6618880, "TC Label"=w457, "PlotColor"=w461, "Temperature"=w460, "Alarm Color"=w458, "Alarm Status"=w459) -> (w456:T7)
                        n209 = property class="WFChart (strict)"(reference=w464, "Plot.Visible?"=TRUE ("Plot.Visible")) -> ()  [unwired: 1 in, 2 out]
                      }
                    }
                  }
                }
                n210 = Replace Array Subset(array=w393, new element=w397, index (row)=w395, index (col)=w394) -> (w399:T3)
                n211 = Bundle By Name(cluster=w400, "Thermocouples"=w399) -> (w392:T6)
              }
            }
          }
          event "Graphing Selection": Value Change {
            n212 = event-data() -> ("NewVal"=w473:u16)  [unwired: 1 in, 5 out]
            n213 = Unbundle By Name(w468) -> ("Thermocouples"=w467:T3, "working array"=w470:bool[])
            n214 = control-ref of="Waveform Chart"() -> (w474:refnum<vi>)
            n215 = case shown="1" w473 {
              tunnel: w467 -> [w475 w480 w511]
              tunnel: w474 -> [_ w479 w510]
              tunnel: 120 ("disabled index (col)") -> [_ w478 w509]
              tunnel: w468 -> [_ _ _]
              tunnel: w470 -> [_ w477 _]
              tunnel: [w475 w476 w508] -> w469
              frame 0, Default {
              }
              frame 1 {
                n216 = for {
                  N: w478 -> [_]
                  tunnel: w479 -> [w486]
                  shift-right: [w481] -> w476
                  shift-left: w480 -> [w485]
                  tunnel: w477 -> [w482]
                  i -> [w484]
                  n217 = Index Array(array=w482, index=w484) -> (element=w483:bool)
                  n218 = case shown="True" w483 {
                    tunnel: w486 -> [_ w507]
                    tunnel: w485 -> [w487 w488]
                    tunnel: [w487 w489] -> w481
                    tunnel: w484 -> [_ w506]
                    frame False {
                    }
                    frame True {
                      n219 = Quotient & Remainder(x=w506, y=4) -> (x-y*floor(x/y)=w492:i32, floor(x/y)=w491:i32)
                      n220 = Multiply(x=4, y=w491) -> (x*y=w502:i32)
                      n221 = Add(x=w502, y=w492) -> (x+y=w501:i32)
                      n222 = property class="WFChart (strict)"(reference=w507, "Active Plot"=w501) -> (reference out=w504:refnum<vi>)  [unwired: 1 in, 1 out]
                      n223 = Index Array(array=w488, index (row)=w491, index (col)=w492) -> (element=w490:T7)
                      n224 = Unbundle By Name(w490) -> ("TC Label"=w493:string, "Alarm Status"=w499:string, "Temperature"=w498:string, "PlotColor"=w495:u32, "Alarm Color"=w494:u32)
                      n225 = property class="WFChart (strict)"(reference=w504, "Plot.Visible?"=TRUE ("Plot.Visible")) -> ()  [unwired: 1 in, 2 out]
                      n226 = Bundle By Name(cluster=w490, "TC Label"=w493, "Alarm Status"=w499, "Alarm Color"=w494, "Temperature"=w498, "PlotColor"=w495, "Graph On/Off"=u32 6618880) -> (w497:T7)
                      n227 = Replace Array Subset(array=w488, new element=w497, index (row)=w491, index (col)=w492) -> (w489:T3)
                    }
                  }
                }
              }
              frame 2 {
                n228 = for {
                  N: w509 -> [_]
                  tunnel: w510 -> [w529]
                  shift-right: [w512] -> w508
                  shift-left: w511 -> [w516]
                  i -> [w530]
                  w522 = u32 12369084
                  n229 = local read "working array"() -> (w531:bool[])
                  n230 = Quotient & Remainder(x=w530, y=4 ("Numeric")) -> (x-y*floor(x/y)=w514:i32, floor(x/y)=w513:i32)
                  n231 = Index Array(array=w516, index (row)=w513, index (col)=w514) -> (element=w521:T7)
                  n232 = Multiply(x=4, y=w513) -> (x*y=w525:i32)
                  n233 = Add(x=w525, y=w514) -> (x+y=w524:i32)
                  n234 = Index Array(array=w531, index=w530) -> ()  [unwired: 1 out]
                  n235 = property class="WFChart (strict)"(reference=w529, "Active Plot"=w524) -> (reference out=w527:refnum<vi>)  [unwired: 1 in, 1 out]
                  n236 = Unbundle By Name(w521) -> ("TC Label"=w520:string, "Alarm Status"=w519:string, "Temperature"=w518:string, "PlotColor"=w517:u32)
                  n237 = property class="WFChart (strict)"(reference=w527, "Plot.Visible?"=FALSE ("Plot.Visible")) -> ()  [unwired: 1 in, 2 out]
                  n238 = Bundle By Name(cluster=w521, "TC Label"=w520, "Alarm Status"=w519, "Alarm Color"=w522, "Temperature"=w518, "PlotColor"=w517, "Graph On/Off"=w522) -> (w515:T7)
                  n239 = Replace Array Subset(array=w516, new element=w515, index (row)=w513, index (col)=w514) -> (w512:T3)
                }
              }
            }
            n240 = Bundle By Name(cluster=w468, "Thermocouples"=w469) -> (w466:T6)
          }
          event "Set Time TC Graph": Mouse Down {
            n241 = event-data() -> ()  [unwired: 1 in, 8 out]
            n242 = local read "Log/Linear Y-Axis"() -> (w533:u16)
            n243 = control-ref of="Waveform Chart"() -> (w532:refnum<vi>)
            n244 = property on="Property Node" class="WFChart (strict)"(reference=w532, "YScale.Mapping Mode"=w533) -> ()  [unwired: 1 in, 2 out]
            n245 = local read "Total Time"() -> (w534:dbl)
            n246 = local read "Time Scale"() -> (w535:u16)
            n247 = case shown="2" w535 {
              tunnel: w532 -> [w540 w559 w578]
              tunnel: w534 -> [w538 w557 w576]
              frame 0, Default {
                n248 = Not Equal To 0?(x=w538) -> (x != 0?=w539:bool)
                n249 = case shown="True" w539 {
                  tunnel: w540 -> [w542 w554]
                  tunnel: w538 -> [_ w548]
                  frame False {
                    n250 = property on="Property Node" class="WFChart (strict)"(reference=w542) -> (reference out=w541:refnum<vi>, "XScale.Range"=w547:T14)  [unwired: 1 in, 1 out]
                    n251 = Bundle By Name(cluster=w547, "Minimum"=0.0, "Maximum"=3600.0, "Increment"=60.0) -> (w546:T14)
                    n252 = property on="Property Node" class="WFChart (strict)"(reference=w541, "XScale.Range"=w546) -> ()  [unwired: 1 in, 2 out]
                  }
                  frame True {
                    n253 = property on="Property Node" class="WFChart (strict)"(reference=w554) -> (reference out=w551:refnum<vi>, "XScale.Range"=w556:T14)  [unwired: 1 in, 1 out]
                    n254 = Multiply(x=w548, y=60.0) -> (x*y=w550:dbl)
                    n255 = Bundle By Name(cluster=w556, "Minimum"=0.0, "Maximum"=w550, "Increment"=1.0) -> (w555:T14)
                    n256 = property on="Property Node" class="WFChart (strict)"(reference=w551, "XScale.Range"=w555) -> ()  [unwired: 1 in, 2 out]
                  }
                }
              }
              frame 1 {
                n257 = Not Equal To 0?(x=w557) -> (x != 0?=w558:bool)
                n258 = case shown="True" w558 {
                  tunnel: w559 -> [w561 w571]
                  tunnel: w557 -> [_ w568]
                  frame False {
                    n259 = property on="Property Node" class="WFChart (strict)"(reference=w561) -> (reference out=w560:refnum<vi>, "XScale.Range"=w566:T14)  [unwired: 1 in, 1 out]
                    n260 = Bundle By Name(cluster=w566, "Minimum"=0.0, "Maximum"=43200.0, "Increment"=3600.0) -> (w562:T14)
                    n261 = property on="Property Node" class="WFChart (strict)"(reference=w560, "XScale.Range"=w562) -> ()  [unwired: 1 in, 2 out]
                  }
                  frame True {
                    n262 = Multiply(x=w568, y=3600.0) -> (x*y=w567:dbl)
                    n263 = property on="Property Node" class="WFChart (strict)"(reference=w571) -> (reference out=w570:refnum<vi>, "XScale.Range"=w575:T14)  [unwired: 1 in, 1 out]
                    n264 = Bundle By Name(cluster=w575, "Minimum"=0.0, "Maximum"=w567, "Increment"=3600.0) -> (w572:T14)
                    n265 = property on="Property Node" class="WFChart (strict)"(reference=w570, "XScale.Range"=w572) -> ()  [unwired: 1 in, 2 out]
                  }
                }
              }
              frame 2 {
                n266 = Not Equal To 0?(x=w576) -> (x != 0?=w577:bool)
                n267 = case shown="True" w577 {
                  tunnel: w578 -> [w580 w588]
                  tunnel: w576 -> [_ w586]
                  frame False {
                    n268 = property on="Property Node" class="WFChart (strict)"(reference=w580) -> (reference out=w579:refnum<vi>, "XScale.Range"=w585:T14)  [unwired: 1 in, 1 out]
                    n269 = Bundle By Name(cluster=w585, "Minimum"=0.0, "Maximum"=60.0, "Increment"=1.0) -> (w581:T14)
                    n270 = property on="Property Node" class="WFChart (strict)"(reference=w579, "XScale.Range"=w581) -> ()  [unwired: 1 in, 2 out]
                  }
                  frame True {
                    n271 = property on="Property Node" class="WFChart (strict)"(reference=w588) -> (reference out=w587:refnum<vi>, "XScale.Range"=w592:T14)  [unwired: 1 in, 1 out]
                    n272 = Bundle By Name(cluster=w592, "Minimum"=0.0, "Maximum"=w586, "Increment"=1.0) -> (w589:T14)
                    n273 = property on="Property Node" class="WFChart (strict)"(reference=w587, "XScale.Range"=w589) -> ()  [unwired: 1 in, 2 out]
                  }
                }
              }
            }
          }
          event "Set Time TC Graph 1": Mouse Down {
            n274 = event-data() -> ()  [unwired: 1 in, 8 out]
            n275 = local read "Log/Linear Y-Axis 1"() -> (w594:u16)
            n276 = control-ref of="Custom Chart 1"() -> (w593:refnum<vi>)
            n277 = property on="Property Node" class="WFChart (strict)"(reference=w593, "YScale.Mapping Mode"=w594) -> ()  [unwired: 1 in, 2 out]
            n278 = local read "Total Time 1"() -> (w595:dbl)
            n279 = local read "Time Scale 1"() -> (w596:u16)
            n280 = case shown="2" w596 {
              tunnel: w593 -> [w601 w620 w639]
              tunnel: w595 -> [w599 w618 w637]
              frame 0, Default {
                n281 = Not Equal To 0?(x=w599) -> (x != 0?=w600:bool)
                n282 = case shown="True" w600 {
                  tunnel: w601 -> [w603 w615]
                  tunnel: w599 -> [_ w609]
                  frame False {
                    n283 = property on="Property Node" class="WFChart (strict)"(reference=w603) -> (reference out=w602:refnum<vi>, "XScale.Range"=w608:T14)  [unwired: 1 in, 1 out]
                    n284 = Bundle By Name(cluster=w608, "Minimum"=0.0, "Maximum"=3600.0, "Increment"=60.0) -> (w607:T14)
                    n285 = property on="Property Node" class="WFChart (strict)"(reference=w602, "XScale.Range"=w607) -> ()  [unwired: 1 in, 2 out]
                  }
                  frame True {
                    n286 = property on="Property Node" class="WFChart (strict)"(reference=w615) -> (reference out=w612:refnum<vi>, "XScale.Range"=w617:T14)  [unwired: 1 in, 1 out]
                    n287 = Multiply(x=w609, y=60.0) -> (x*y=w611:dbl)
                    n288 = Bundle By Name(cluster=w617, "Minimum"=0.0, "Maximum"=w611, "Increment"=1.0) -> (w616:T14)
                    n289 = property on="Property Node" class="WFChart (strict)"(reference=w612, "XScale.Range"=w616) -> ()  [unwired: 1 in, 2 out]
                  }
                }
              }
              frame 1 {
                n290 = Not Equal To 0?(x=w618) -> (x != 0?=w619:bool)
                n291 = case shown="True" w619 {
                  tunnel: w620 -> [w622 w632]
                  tunnel: w618 -> [_ w629]
                  frame False {
                    n292 = property on="Property Node" class="WFChart (strict)"(reference=w622) -> (reference out=w621:refnum<vi>, "XScale.Range"=w627:T14)  [unwired: 1 in, 1 out]
                    n293 = Bundle By Name(cluster=w627, "Minimum"=0.0, "Maximum"=43200.0, "Increment"=3600.0) -> (w623:T14)
                    n294 = property on="Property Node" class="WFChart (strict)"(reference=w621, "XScale.Range"=w623) -> ()  [unwired: 1 in, 2 out]
                  }
                  frame True {
                    n295 = Multiply(x=w629, y=3600.0) -> (x*y=w628:dbl)
                    n296 = property on="Property Node" class="WFChart (strict)"(reference=w632) -> (reference out=w631:refnum<vi>, "XScale.Range"=w636:T14)  [unwired: 1 in, 1 out]
                    n297 = Bundle By Name(cluster=w636, "Minimum"=0.0, "Maximum"=w628, "Increment"=3600.0) -> (w633:T14)
                    n298 = property on="Property Node" class="WFChart (strict)"(reference=w631, "XScale.Range"=w633) -> ()  [unwired: 1 in, 2 out]
                  }
                }
              }
              frame 2 {
                n299 = Not Equal To 0?(x=w637) -> (x != 0?=w638:bool)
                n300 = case shown="True" w638 {
                  tunnel: w639 -> [w641 w649]
                  tunnel: w637 -> [_ w647]
                  frame False {
                    n301 = property on="Property Node" class="WFChart (strict)"(reference=w641) -> (reference out=w640:refnum<vi>, "XScale.Range"=w646:T14)  [unwired: 1 in, 1 out]
                    n302 = Bundle By Name(cluster=w646, "Minimum"=0.0, "Maximum"=60.0, "Increment"=1.0) -> (w642:T14)
                    n303 = property on="Property Node" class="WFChart (strict)"(reference=w640, "XScale.Range"=w642) -> ()  [unwired: 1 in, 2 out]
                  }
                  frame True {
                    n304 = property on="Property Node" class="WFChart (strict)"(reference=w649) -> (reference out=w648:refnum<vi>, "XScale.Range"=w653:T14)  [unwired: 1 in, 1 out]
                    n305 = Bundle By Name(cluster=w653, "Minimum"=0.0, "Maximum"=w647, "Increment"=1.0) -> (w650:T14)
                    n306 = property on="Property Node" class="WFChart (strict)"(reference=w648, "XScale.Range"=w650) -> ()  [unwired: 1 in, 2 out]
                  }
                }
              }
            }
          }
          event "Set Time TC Graph 2": Mouse Down {
            n307 = event-data() -> ()  [unwired: 1 in, 8 out]
            n308 = local read "Log/Linear Y-Axis 2"() -> (w655:u16)
            n309 = control-ref of="Custom Chart 2"() -> (w654:refnum<vi>)
            n310 = property on="Property Node" class="WFChart (strict)"(reference=w654, "YScale.Mapping Mode"=w655) -> ()  [unwired: 1 in, 2 out]
            n311 = local read "Total Time 2"() -> (w656:dbl)
            n312 = local read "Time Scale 2"() -> (w657:u16)
            n313 = case shown="2" w657 {
              tunnel: w654 -> [w662 w681 w700]
              tunnel: w656 -> [w660 w679 w698]
              frame 0, Default {
                n314 = Not Equal To 0?(x=w660) -> (x != 0?=w661:bool)
                n315 = case shown="True" w661 {
                  tunnel: w662 -> [w664 w676]
                  tunnel: w660 -> [_ w670]
                  frame False {
                    n316 = property on="Property Node" class="WFChart (strict)"(reference=w664) -> (reference out=w663:refnum<vi>, "XScale.Range"=w669:T14)  [unwired: 1 in, 1 out]
                    n317 = Bundle By Name(cluster=w669, "Minimum"=0.0, "Maximum"=3600.0, "Increment"=60.0) -> (w668:T14)
                    n318 = property on="Property Node" class="WFChart (strict)"(reference=w663, "XScale.Range"=w668) -> ()  [unwired: 1 in, 2 out]
                  }
                  frame True {
                    n319 = property on="Property Node" class="WFChart (strict)"(reference=w676) -> (reference out=w673:refnum<vi>, "XScale.Range"=w678:T14)  [unwired: 1 in, 1 out]
                    n320 = Multiply(x=w670, y=60.0) -> (x*y=w672:dbl)
                    n321 = Bundle By Name(cluster=w678, "Minimum"=0.0, "Maximum"=w672, "Increment"=1.0) -> (w677:T14)
                    n322 = property on="Property Node" class="WFChart (strict)"(reference=w673, "XScale.Range"=w677) -> ()  [unwired: 1 in, 2 out]
                  }
                }
              }
              frame 1 {
                n323 = Not Equal To 0?(x=w679) -> (x != 0?=w680:bool)
                n324 = case shown="True" w680 {
                  tunnel: w681 -> [w683 w693]
                  tunnel: w679 -> [_ w690]
                  frame False {
                    n325 = property on="Property Node" class="WFChart (strict)"(reference=w683) -> (reference out=w682:refnum<vi>, "XScale.Range"=w688:T14)  [unwired: 1 in, 1 out]
                    n326 = Bundle By Name(cluster=w688, "Minimum"=0.0, "Maximum"=43200.0, "Increment"=3600.0) -> (w684:T14)
                    n327 = property on="Property Node" class="WFChart (strict)"(reference=w682, "XScale.Range"=w684) -> ()  [unwired: 1 in, 2 out]
                  }
                  frame True {
                    n328 = Multiply(x=w690, y=3600.0) -> (x*y=w689:dbl)
                    n329 = property on="Property Node" class="WFChart (strict)"(reference=w693) -> (reference out=w692:refnum<vi>, "XScale.Range"=w697:T14)  [unwired: 1 in, 1 out]
                    n330 = Bundle By Name(cluster=w697, "Minimum"=0.0, "Maximum"=w689, "Increment"=3600.0) -> (w694:T14)
                    n331 = property on="Property Node" class="WFChart (strict)"(reference=w692, "XScale.Range"=w694) -> ()  [unwired: 1 in, 2 out]
                  }
                }
              }
              frame 2 {
                n332 = Not Equal To 0?(x=w698) -> (x != 0?=w699:bool)
                n333 = case shown="True" w699 {
                  tunnel: w700 -> [w702 w710]
                  tunnel: w698 -> [_ w708]
                  frame False {
                    n334 = property on="Property Node" class="WFChart (strict)"(reference=w702) -> (reference out=w701:refnum<vi>, "XScale.Range"=w707:T14)  [unwired: 1 in, 1 out]
                    n335 = Bundle By Name(cluster=w707, "Minimum"=0.0, "Maximum"=60.0, "Increment"=1.0) -> (w703:T14)
                    n336 = property on="Property Node" class="WFChart (strict)"(reference=w701, "XScale.Range"=w703) -> ()  [unwired: 1 in, 2 out]
                  }
                  frame True {
                    n337 = property on="Property Node" class="WFChart (strict)"(reference=w710) -> (reference out=w709:refnum<vi>, "XScale.Range"=w714:T14)  [unwired: 1 in, 1 out]
                    n338 = Bundle By Name(cluster=w714, "Minimum"=0.0, "Maximum"=w708, "Increment"=1.0) -> (w711:T14)
                    n339 = property on="Property Node" class="WFChart (strict)"(reference=w709, "XScale.Range"=w711) -> ()  [unwired: 1 in, 2 out]
                  }
                }
              }
            }
          }
          event "Set Time TC Graph 3": Mouse Down {
            n340 = event-data() -> ()  [unwired: 1 in, 8 out]
            n341 = local read "Log/Linear Y-Axis 3"() -> (w716:u16)
            n342 = control-ref of="Custom Chart 3"() -> (w715:refnum<vi>)
            n343 = property on="Property Node" class="WFChart (strict)"(reference=w715, "YScale.Mapping Mode"=w716) -> ()  [unwired: 1 in, 2 out]
            n344 = local read "Total Time 3"() -> (w717:dbl)
            n345 = local read "Time Scale 3"() -> (w718:u16)
            n346 = case shown="2" w718 {
              tunnel: w715 -> [w723 w742 w761]
              tunnel: w717 -> [w721 w740 w759]
              frame 0, Default {
                n347 = Not Equal To 0?(x=w721) -> (x != 0?=w722:bool)
                n348 = case shown="True" w722 {
                  tunnel: w723 -> [w725 w737]
                  tunnel: w721 -> [_ w731]
                  frame False {
                    n349 = property on="Property Node" class="WFChart (strict)"(reference=w725) -> (reference out=w724:refnum<vi>, "XScale.Range"=w730:T14)  [unwired: 1 in, 1 out]
                    n350 = Bundle By Name(cluster=w730, "Minimum"=0.0, "Maximum"=3600.0, "Increment"=60.0) -> (w729:T14)
                    n351 = property on="Property Node" class="WFChart (strict)"(reference=w724, "XScale.Range"=w729) -> ()  [unwired: 1 in, 2 out]
                  }
                  frame True {
                    n352 = property on="Property Node" class="WFChart (strict)"(reference=w737) -> (reference out=w734:refnum<vi>, "XScale.Range"=w739:T14)  [unwired: 1 in, 1 out]
                    n353 = Multiply(x=w731, y=60.0) -> (x*y=w733:dbl)
                    n354 = Bundle By Name(cluster=w739, "Minimum"=0.0, "Maximum"=w733, "Increment"=1.0) -> (w738:T14)
                    n355 = property on="Property Node" class="WFChart (strict)"(reference=w734, "XScale.Range"=w738) -> ()  [unwired: 1 in, 2 out]
                  }
                }
              }
              frame 1 {
                n356 = Not Equal To 0?(x=w740) -> (x != 0?=w741:bool)
                n357 = case shown="True" w741 {
                  tunnel: w742 -> [w744 w754]
                  tunnel: w740 -> [_ w751]
                  frame False {
                    n358 = property on="Property Node" class="WFChart (strict)"(reference=w744) -> (reference out=w743:refnum<vi>, "XScale.Range"=w749:T14)  [unwired: 1 in, 1 out]
                    n359 = Bundle By Name(cluster=w749, "Minimum"=0.0, "Maximum"=43200.0, "Increment"=3600.0) -> (w745:T14)
                    n360 = property on="Property Node" class="WFChart (strict)"(reference=w743, "XScale.Range"=w745) -> ()  [unwired: 1 in, 2 out]
                  }
                  frame True {
                    n361 = Multiply(x=w751, y=3600.0) -> (x*y=w750:dbl)
                    n362 = property on="Property Node" class="WFChart (strict)"(reference=w754) -> (reference out=w753:refnum<vi>, "XScale.Range"=w758:T14)  [unwired: 1 in, 1 out]
                    n363 = Bundle By Name(cluster=w758, "Minimum"=0.0, "Maximum"=w750, "Increment"=3600.0) -> (w755:T14)
                    n364 = property on="Property Node" class="WFChart (strict)"(reference=w753, "XScale.Range"=w755) -> ()  [unwired: 1 in, 2 out]
                  }
                }
              }
              frame 2 {
                n365 = Not Equal To 0?(x=w759) -> (x != 0?=w760:bool)
                n366 = case shown="True" w760 {
                  tunnel: w761 -> [w763 w771]
                  tunnel: w759 -> [_ w769]
                  frame False {
                    n367 = property on="Property Node" class="WFChart (strict)"(reference=w763) -> (reference out=w762:refnum<vi>, "XScale.Range"=w768:T14)  [unwired: 1 in, 1 out]
                    n368 = Bundle By Name(cluster=w768, "Minimum"=0.0, "Maximum"=60.0, "Increment"=1.0) -> (w764:T14)
                    n369 = property on="Property Node" class="WFChart (strict)"(reference=w762, "XScale.Range"=w764) -> ()  [unwired: 1 in, 2 out]
                  }
                  frame True {
                    n370 = property on="Property Node" class="WFChart (strict)"(reference=w771) -> (reference out=w770:refnum<vi>, "XScale.Range"=w775:T14)  [unwired: 1 in, 1 out]
                    n371 = Bundle By Name(cluster=w775, "Minimum"=0.0, "Maximum"=w769, "Increment"=1.0) -> (w772:T14)
                    n372 = property on="Property Node" class="WFChart (strict)"(reference=w770, "XScale.Range"=w772) -> ()  [unwired: 1 in, 2 out]
                  }
                }
              }
            }
          }
          event "Set Time TC Graph 4": Mouse Down {
            n373 = event-data() -> ()  [unwired: 1 in, 8 out]
            n374 = local read "Log/Linear Y-Axis 4"() -> (w777:u16)
            n375 = control-ref of="Custom Chart 4"() -> (w776:refnum<vi>)
            n376 = property on="Property Node" class="WFChart (strict)"(reference=w776, "YScale.Mapping Mode"=w777) -> ()  [unwired: 1 in, 2 out]
            n377 = local read "Total Time 4"() -> (w778:dbl)
            n378 = local read "Time Scale 4"() -> (w779:u16)
            n379 = case shown="2" w779 {
              tunnel: w776 -> [w784 w803 w822]
              tunnel: w778 -> [w782 w801 w820]
              frame 0, Default {
                n380 = Not Equal To 0?(x=w782) -> (x != 0?=w783:bool)
                n381 = case shown="True" w783 {
                  tunnel: w784 -> [w786 w798]
                  tunnel: w782 -> [_ w792]
                  frame False {
                    n382 = property on="Property Node" class="WFChart (strict)"(reference=w786) -> (reference out=w785:refnum<vi>, "XScale.Range"=w791:T14)  [unwired: 1 in, 1 out]
                    n383 = Bundle By Name(cluster=w791, "Minimum"=0.0, "Maximum"=3600.0, "Increment"=60.0) -> (w790:T14)
                    n384 = property on="Property Node" class="WFChart (strict)"(reference=w785, "XScale.Range"=w790) -> ()  [unwired: 1 in, 2 out]
                  }
                  frame True {
                    n385 = property on="Property Node" class="WFChart (strict)"(reference=w798) -> (reference out=w795:refnum<vi>, "XScale.Range"=w800:T14)  [unwired: 1 in, 1 out]
                    n386 = Multiply(x=w792, y=60.0) -> (x*y=w794:dbl)
                    n387 = Bundle By Name(cluster=w800, "Minimum"=0.0, "Maximum"=w794, "Increment"=1.0) -> (w799:T14)
                    n388 = property on="Property Node" class="WFChart (strict)"(reference=w795, "XScale.Range"=w799) -> ()  [unwired: 1 in, 2 out]
                  }
                }
              }
              frame 1 {
                n389 = Not Equal To 0?(x=w801) -> (x != 0?=w802:bool)
                n390 = case shown="True" w802 {
                  tunnel: w803 -> [w805 w815]
                  tunnel: w801 -> [_ w812]
                  frame False {
                    n391 = property on="Property Node" class="WFChart (strict)"(reference=w805) -> (reference out=w804:refnum<vi>, "XScale.Range"=w810:T14)  [unwired: 1 in, 1 out]
                    n392 = Bundle By Name(cluster=w810, "Minimum"=0.0, "Maximum"=43200.0, "Increment"=3600.0) -> (w806:T14)
                    n393 = property on="Property Node" class="WFChart (strict)"(reference=w804, "XScale.Range"=w806) -> ()  [unwired: 1 in, 2 out]
                  }
                  frame True {
                    n394 = Multiply(x=w812, y=3600.0) -> (x*y=w811:dbl)
                    n395 = property on="Property Node" class="WFChart (strict)"(reference=w815) -> (reference out=w814:refnum<vi>, "XScale.Range"=w819:T14)  [unwired: 1 in, 1 out]
                    n396 = Bundle By Name(cluster=w819, "Minimum"=0.0, "Maximum"=w811, "Increment"=3600.0) -> (w816:T14)
                    n397 = property on="Property Node" class="WFChart (strict)"(reference=w814, "XScale.Range"=w816) -> ()  [unwired: 1 in, 2 out]
                  }
                }
              }
              frame 2 {
                n398 = Not Equal To 0?(x=w820) -> (x != 0?=w821:bool)
                n399 = case shown="True" w821 {
                  tunnel: w822 -> [w824 w832]
                  tunnel: w820 -> [_ w830]
                  frame False {
                    n400 = property on="Property Node" class="WFChart (strict)"(reference=w824) -> (reference out=w823:refnum<vi>, "XScale.Range"=w829:T14)  [unwired: 1 in, 1 out]
                    n401 = Bundle By Name(cluster=w829, "Minimum"=0.0, "Maximum"=60.0, "Increment"=1.0) -> (w825:T14)
                    n402 = property on="Property Node" class="WFChart (strict)"(reference=w823, "XScale.Range"=w825) -> ()  [unwired: 1 in, 2 out]
                  }
                  frame True {
                    n403 = property on="Property Node" class="WFChart (strict)"(reference=w832) -> (reference out=w831:refnum<vi>, "XScale.Range"=w836:T14)  [unwired: 1 in, 1 out]
                    n404 = Bundle By Name(cluster=w836, "Minimum"=0.0, "Maximum"=w830, "Increment"=1.0) -> (w833:T14)
                    n405 = property on="Property Node" class="WFChart (strict)"(reference=w831, "XScale.Range"=w833) -> ()  [unwired: 1 in, 2 out]
                  }
                }
              }
            }
          }
          event "Set Time TC Graph 5": Mouse Down {
            n406 = event-data() -> ()  [unwired: 1 in, 8 out]
            n407 = local read "Log/Linear Y-Axis 5"() -> (w838:u16)
            n408 = control-ref of="Custom Chart 5"() -> (w837:refnum<vi>)
            n409 = property on="Property Node" class="WFChart (strict)"(reference=w837, "YScale.Mapping Mode"=w838) -> ()  [unwired: 1 in, 2 out]
            n410 = local read "Total Time 5"() -> (w839:dbl)
            n411 = local read "Time Scale 5"() -> (w840:u16)
            n412 = case shown="2" w840 {
              tunnel: w837 -> [w845 w864 w883]
              tunnel: w839 -> [w843 w862 w881]
              frame 0, Default {
                n413 = Not Equal To 0?(x=w843) -> (x != 0?=w844:bool)
                n414 = case shown="True" w844 {
                  tunnel: w845 -> [w847 w859]
                  tunnel: w843 -> [_ w853]
                  frame False {
                    n415 = property on="Property Node" class="WFChart (strict)"(reference=w847) -> (reference out=w846:refnum<vi>, "XScale.Range"=w852:T14)  [unwired: 1 in, 1 out]
                    n416 = Bundle By Name(cluster=w852, "Minimum"=0.0, "Maximum"=3600.0, "Increment"=60.0) -> (w851:T14)
                    n417 = property on="Property Node" class="WFChart (strict)"(reference=w846, "XScale.Range"=w851) -> ()  [unwired: 1 in, 2 out]
                  }
                  frame True {
                    n418 = property on="Property Node" class="WFChart (strict)"(reference=w859) -> (reference out=w856:refnum<vi>, "XScale.Range"=w861:T14)  [unwired: 1 in, 1 out]
                    n419 = Multiply(x=w853, y=60.0) -> (x*y=w855:dbl)
                    n420 = Bundle By Name(cluster=w861, "Minimum"=0.0, "Maximum"=w855, "Increment"=1.0) -> (w860:T14)
                    n421 = property on="Property Node" class="WFChart (strict)"(reference=w856, "XScale.Range"=w860) -> ()  [unwired: 1 in, 2 out]
                  }
                }
              }
              frame 1 {
                n422 = Not Equal To 0?(x=w862) -> (x != 0?=w863:bool)
                n423 = case shown="True" w863 {
                  tunnel: w864 -> [w866 w876]
                  tunnel: w862 -> [_ w873]
                  frame False {
                    n424 = property on="Property Node" class="WFChart (strict)"(reference=w866) -> (reference out=w865:refnum<vi>, "XScale.Range"=w871:T14)  [unwired: 1 in, 1 out]
                    n425 = Bundle By Name(cluster=w871, "Minimum"=0.0, "Maximum"=43200.0, "Increment"=3600.0) -> (w867:T14)
                    n426 = property on="Property Node" class="WFChart (strict)"(reference=w865, "XScale.Range"=w867) -> ()  [unwired: 1 in, 2 out]
                  }
                  frame True {
                    n427 = Multiply(x=w873, y=3600.0) -> (x*y=w872:dbl)
                    n428 = property on="Property Node" class="WFChart (strict)"(reference=w876) -> (reference out=w875:refnum<vi>, "XScale.Range"=w880:T14)  [unwired: 1 in, 1 out]
                    n429 = Bundle By Name(cluster=w880, "Minimum"=0.0, "Maximum"=w872, "Increment"=3600.0) -> (w877:T14)
                    n430 = property on="Property Node" class="WFChart (strict)"(reference=w875, "XScale.Range"=w877) -> ()  [unwired: 1 in, 2 out]
                  }
                }
              }
              frame 2 {
                n431 = Not Equal To 0?(x=w881) -> (x != 0?=w882:bool)
                n432 = case shown="True" w882 {
                  tunnel: w883 -> [w885 w893]
                  tunnel: w881 -> [_ w891]
                  frame False {
                    n433 = property on="Property Node" class="WFChart (strict)"(reference=w885) -> (reference out=w884:refnum<vi>, "XScale.Range"=w890:T14)  [unwired: 1 in, 1 out]
                    n434 = Bundle By Name(cluster=w890, "Minimum"=0.0, "Maximum"=60.0, "Increment"=1.0) -> (w886:T14)
                    n435 = property on="Property Node" class="WFChart (strict)"(reference=w884, "XScale.Range"=w886) -> ()  [unwired: 1 in, 2 out]
                  }
                  frame True {
                    n436 = property on="Property Node" class="WFChart (strict)"(reference=w893) -> (reference out=w892:refnum<vi>, "XScale.Range"=w897:T14)  [unwired: 1 in, 1 out]
                    n437 = Bundle By Name(cluster=w897, "Minimum"=0.0, "Maximum"=w891, "Increment"=1.0) -> (w894:T14)
                    n438 = property on="Property Node" class="WFChart (strict)"(reference=w892, "XScale.Range"=w894) -> ()  [unwired: 1 in, 2 out]
                  }
                }
              }
            }
          }
          event "Set Time TC Graph 6": Mouse Down {
            n439 = event-data() -> ()  [unwired: 1 in, 8 out]
            n440 = local read "Log/Linear Y-Axis 6"() -> (w899:u16)
            n441 = control-ref of="Custom Chart 6"() -> (w898:refnum<vi>)
            n442 = property on="Property Node" class="WFChart (strict)"(reference=w898, "YScale.Mapping Mode"=w899) -> ()  [unwired: 1 in, 2 out]
            n443 = local read "Total Time 6"() -> (w900:dbl)
            n444 = local read "Time Scale 6"() -> (w901:u16)
            n445 = case shown="2" w901 {
              tunnel: w898 -> [w906 w925 w944]
              tunnel: w900 -> [w904 w923 w942]
              frame 0, Default {
                n446 = Not Equal To 0?(x=w904) -> (x != 0?=w905:bool)
                n447 = case shown="True" w905 {
                  tunnel: w906 -> [w908 w920]
                  tunnel: w904 -> [_ w914]
                  frame False {
                    n448 = property on="Property Node" class="WFChart (strict)"(reference=w908) -> (reference out=w907:refnum<vi>, "XScale.Range"=w913:T14)  [unwired: 1 in, 1 out]
                    n449 = Bundle By Name(cluster=w913, "Minimum"=0.0, "Maximum"=3600.0, "Increment"=60.0) -> (w912:T14)
                    n450 = property on="Property Node" class="WFChart (strict)"(reference=w907, "XScale.Range"=w912) -> ()  [unwired: 1 in, 2 out]
                  }
                  frame True {
                    n451 = property on="Property Node" class="WFChart (strict)"(reference=w920) -> (reference out=w917:refnum<vi>, "XScale.Range"=w922:T14)  [unwired: 1 in, 1 out]
                    n452 = Multiply(x=w914, y=60.0) -> (x*y=w916:dbl)
                    n453 = Bundle By Name(cluster=w922, "Minimum"=0.0, "Maximum"=w916, "Increment"=1.0) -> (w921:T14)
                    n454 = property on="Property Node" class="WFChart (strict)"(reference=w917, "XScale.Range"=w921) -> ()  [unwired: 1 in, 2 out]
                  }
                }
              }
              frame 1 {
                n455 = Not Equal To 0?(x=w923) -> (x != 0?=w924:bool)
                n456 = case shown="True" w924 {
                  tunnel: w925 -> [w927 w937]
                  tunnel: w923 -> [_ w934]
                  frame False {
                    n457 = property on="Property Node" class="WFChart (strict)"(reference=w927) -> (reference out=w926:refnum<vi>, "XScale.Range"=w932:T14)  [unwired: 1 in, 1 out]
                    n458 = Bundle By Name(cluster=w932, "Minimum"=0.0, "Maximum"=43200.0, "Increment"=3600.0) -> (w928:T14)
                    n459 = property on="Property Node" class="WFChart (strict)"(reference=w926, "XScale.Range"=w928) -> ()  [unwired: 1 in, 2 out]
                  }
                  frame True {
                    n460 = Multiply(x=w934, y=3600.0) -> (x*y=w933:dbl)
                    n461 = property on="Property Node" class="WFChart (strict)"(reference=w937) -> (reference out=w936:refnum<vi>, "XScale.Range"=w941:T14)  [unwired: 1 in, 1 out]
                    n462 = Bundle By Name(cluster=w941, "Minimum"=0.0, "Maximum"=w933, "Increment"=3600.0) -> (w938:T14)
                    n463 = property on="Property Node" class="WFChart (strict)"(reference=w936, "XScale.Range"=w938) -> ()  [unwired: 1 in, 2 out]
                  }
                }
              }
              frame 2 {
                n464 = Not Equal To 0?(x=w942) -> (x != 0?=w943:bool)
                n465 = case shown="True" w943 {
                  tunnel: w944 -> [w946 w954]
                  tunnel: w942 -> [_ w952]
                  frame False {
                    n466 = property on="Property Node" class="WFChart (strict)"(reference=w946) -> (reference out=w945:refnum<vi>, "XScale.Range"=w951:T14)  [unwired: 1 in, 1 out]
                    n467 = Bundle By Name(cluster=w951, "Minimum"=0.0, "Maximum"=60.0, "Increment"=1.0) -> (w947:T14)
                    n468 = property on="Property Node" class="WFChart (strict)"(reference=w945, "XScale.Range"=w947) -> ()  [unwired: 1 in, 2 out]
                  }
                  frame True {
                    n469 = property on="Property Node" class="WFChart (strict)"(reference=w954) -> (reference out=w953:refnum<vi>, "XScale.Range"=w958:T14)  [unwired: 1 in, 1 out]
                    n470 = Bundle By Name(cluster=w958, "Minimum"=0.0, "Maximum"=w952, "Increment"=1.0) -> (w955:T14)
                    n471 = property on="Property Node" class="WFChart (strict)"(reference=w953, "XScale.Range"=w955) -> ()  [unwired: 1 in, 2 out]
                  }
                }
              }
            }
          }
          event "exit": Value Change {
            n472 = event-data() -> ()  [unwired: 1 in, 1 out]
            n473 = call "Deliver Message.vi"("error in (no error)"=w961, "event"="exit") -> ("error out"=w959:errorcluster)  [unwired: 9 in]
          }
        }
      }
      frame "getPressure" {
        n474 = Unbundle By Name(w968) -> ("Http session"=w977:T5, "URL prefex"=w975:string)
        n475 = local read "Local Debug"() -> (w963:bool)
        n476 = Build Array(3, 2, 1) -> (w973:i32[])
        n477 = Flatten To JSON(anything=w973) -> (JSON string=w972:string)  [unwired: 2 in, 1 out]
        n478 = Concatenate Strings(w975, "getPressureGauges" ("url")) -> (w976:string)
        n479 = case shown="False" w963 {
          tunnel: [w983 w999] -> w978
          tunnel: w977 -> [w983 w998]
          tunnel: w976 -> [w981 w997]
          tunnel: w972 -> [_ w996]
          tunnel: w967 -> [w982 w994]
          tunnel: [w982 w993] -> w966
          tunnel: [w980 w992] -> w964
          frame False {
            n480 = case shown="True" "read pressure" {
              tunnel: w981 -> [_ w991]
              tunnel: [_ w984] -> w980
              frame False {
              }
              frame True {
                n481 = call <vilib>:"GET.vi"("url"=w991) -> ("body"=w986:string)  [unwired: 11 in, 3 out]
                n482 = Unflatten From JSON(JSON string=w986, type and defaults=T8 {"CryoPressure"=0.0, "ChamberPressure"=0.0, "RoughingPressure"=0.0}) -> (value=w990:T8)  [unwired: 5 in, 1 out]
                n483 = Unbundle By Name(w990) -> ("CryoPressure"=w989:dbl, "ChamberPressure"=w988:dbl, "RoughingPressure"=w987:dbl)
                n484 = Build Array(w989, w988, w987) -> (w984:dbl[])
              }
            }
          }
          frame True {
            n485 = call-poly <vilib>:"POST.vi"("client handle"=w998, "url"=w997, "buffer"=w996, "error in (no error)"=w994) -> ("client handle out"=w999:T5, "body"=w995:string, "error out"=w993:errorcluster)  [unwired: 8 in, 1 out]
            n486 = case shown="Default" w995 {
              selector: w995 -> [_ w1005 w1007]
              tunnel: [_ w1000 _] -> w992
              frame "" {
              }
              frame Default {
                n487 = Unflatten From JSON(JSON string=w1005, type and defaults=T8 {"CryoPressure"=0.0, "ChamberPressure"=0.0, "RoughingPressure"=0.0}) -> (value=w1004:T8)  [unwired: 5 in, 1 out]
                n488 = Unbundle By Name(w1004) -> ("CryoPressure"=w1003:dbl, "ChamberPressure"=w1002:dbl, "RoughingPressure"=w1001:dbl)
                n489 = Build Array(w1003, w1002, w1001) -> (w1000:dbl[])
              }
              frame "Buffer Needs to be list" {
                n490 = One Button Dialog(message=w1007) -> ()  [unwired: 1 in, 1 out]
              }
            }
          }
        }
        n491 = Bundle By Name(cluster=w968, "Http session"=w978, "Pressure"=w964) -> (w965:T6)
      }
      frame "getTC" {
        w1025 = T10 {"time"="", "TCs"=[]} ("Cluster")
        n492 = property on="Waveform Chart" class="WFChart (strict)"("LegScrollVis"=TRUE ("Legend:Scrollbar Visible")) -> ()  [unwired: 2 in, 2 out]
        n493 = local read "Local Debug"() -> (w1023:bool)
        n494 = Unbundle By Name(w1018) -> ("Http session"=w1032:T5, "URL prefex"=w1030:string)
        n495 = Concatenate Strings(w1030, "getAllThermoCoupleData" ("url")) -> (w1031:string)
        n496 = Flatten To JSON(anything=w1025) -> (JSON string=w1024:string)  [unwired: 2 in, 1 out]
        n497 = case shown="True" w1023 {
          tunnel: w1034 -> [w1107 w1108]
          tunnel: [w1106 w1109] -> w1008
          tunnel: [w1105 w1110] -> w1033
          tunnel: w1032 -> [w1104 w1113]
          tunnel: w1031 -> [w1103 w1114]
          tunnel: [w1102 w1111] -> w1028
          tunnel: [w1101 w1112] -> _
          tunnel: w1024 -> [_ w1115]
          frame False {
            n498 = call <vilib>:"GET.vi"("client handle"=w1104, "url"=w1103, "error in (no error)"=w1107) -> ("client handle out"=w1105:T5, "headers"=w1101:string, "body"=w1102:string, "error out"=w1106:errorcluster)  [unwired: 9 in]
          }
          frame True {
            n499 = call-poly <vilib>:"POST.vi"("client handle"=w1113, "url"=w1114, "buffer"=w1115, "error in (no error)"=w1108) -> ("client handle out"=w1110:T5, "headers"=w1112:string, "body"=w1111:string, "error out"=w1109:errorcluster)  [unwired: 8 in]
          }
        }
        n500 = Bundle By Name(cluster=w1018, "Http session"=w1033) -> (w1022:T6)
        n501 = Unflatten From JSON(JSON string=w1028, type and defaults=w1025) -> (value=w1027:T10)  [unwired: 5 in, 1 out]
        n502 = Unbundle By Name(w1027) -> ("TCs"=w1014:T11)
        n503 = Unbundle By Name(w1022) -> ("working array"=w1015:bool[], "Thermocouples"=w1016:T3)
        n504 = for {
          N: 120 -> [_]
          tunnel: w1014 -> [w1064] mode=indexing
          tunnel: [w1063] -> w1009 mode=indexing
          shift-right: [w1042] -> w1011
          shift-left: w1016 -> [w1049]
          shift-right: [w1041] -> w1017
          shift-left: w1015 -> [w1040]
          i -> [w1039]
          n505 = Unbundle By Name(w1064) -> ("thermocouple"=w1073:i32, "temp"=w1037:dbl, "alarm"=w1068:i32, "working"=w1067:bool)
          n506 = Quotient & Remainder(x=w1039, y=4) -> (x-y*floor(x/y)=w1047:i32, floor(x/y)=w1048:i32)
          n507 = Index Array(array=w1049, index (row)=w1048, index (col)=w1047) -> (element=w1062:T7)
          n508 = Multiply(x=w1048, y=4) -> (x*y=w1057:i32)
          n509 = Multiply(x=w1048, y=4) -> (x*y=w1069:i32)
          n510 = Unbundle By Name(w1062) -> ("Graph On/Off"=w1046:u32)
          n511 = Add(x=w1057, y=w1047) -> (x+y=w1055:i32)
          n512 = Add(x=w1069, y=w1047) -> (x+y=w1038:i32)
          n513 = Replace Array Subset(array=w1040, new element=w1067, index=w1039) -> (w1041:bool[])
          n514 = To Double Precision Float(number=w1037) -> (double precision float=w1036:dbl)
          n515 = Get Date/Time In Seconds() -> (seconds since 1Jan1904=w1066:timestamp)
          n516 = property on="Waveform Chart" class="WFChart (strict)"("Active Plot"=w1038) -> ()  [unwired: 2 in, 2 out]
          n517 = Index Array(array=w1041, index=w1055) -> (element=w1054:bool)
          n518 = Bundle By Name("t0"=w1066) -> (w1065:waveform(dbl))  [unwired: 1 in]
          n519 = Build Array(w1036) -> (w1035:dbl[])
          n520 = Number To Fractional String(number=w1036, precision (6)=i16 2 ("width (-)")) -> (F-format string=w1052:string)  [unwired: 2 in]
          n521 = Bundle By Name(cluster=w1065, "Y"=w1035) -> (w1063:waveform(dbl))
          n522 = case shown="True" w1054 {
            tunnel: w1046 -> [_ w1078]
            tunnel: [u32 12369084 ("y") w1078] -> w1050
            tunnel: w1052 -> [_ w1077]
            tunnel: ["NaN" w1077] -> w1051
            frame False {
            }
            frame True {
            }
          }
          n523 = case shown="1" w1068 {
            tunnel: ["" "L" "H"] -> w1043
            tunnel: w1068 -> [_ _ _]
            tunnel: [u32 12369084 u32 2812927 u32 16711680] -> w1044
            frame 0, Default {
            }
            frame 1 {
            }
            frame 2 {
            }
          }
          n524 = Number To Decimal String(number=w1073) -> (decimal integer string=w1074:string)  [unwired: 1 in]
          n525 = Index Array(array=w1049, index (row)=w1048, index (col)=w1047) -> (element=w1060:T7)
          n526 = Equal?(x=w1050, y=u32 6618880) -> (x = y?=w1058:bool)
          n527 = Concatenate Strings("TC " ("string"), w1074) -> (w1045:string)
          n528 = property on="Waveform Chart" class="WFChart (strict)"("Plot.Plot Name"=w1045) -> ()  [unwired: 2 in, 2 out]
          n529 = case shown="True" w1058 {
            tunnel: [w1086 w1094] -> w1061
            tunnel: w1060 -> [w1085 w1093]
            tunnel: w1050 -> [w1083 w1092]
            tunnel: w1051 -> [w1084 w1091]
            tunnel: w1045 -> [w1082 w1090]
            tunnel: w1044 -> [w1081 w1089]
            tunnel: w1043 -> [w1080 w1088]
            frame False {
              n530 = Bundle By Name(cluster=w1085, "Graph On/Off"=w1083, "TC Label"=w1082, "PlotColor"=u32 12369084 ("y"), "Temperature"=w1084, "Alarm Color"=w1081, "Alarm Status"=w1080) -> (w1086:T7)
            }
            frame True {
              n531 = property on="Waveform Chart" class="WFChart (strict)"() -> ("Plot.Plot Color"=w1087:u32)  [unwired: 2 in, 2 out]
              n532 = Bundle By Name(cluster=w1093, "Graph On/Off"=w1092, "TC Label"=w1090, "PlotColor"=w1087, "Temperature"=w1091, "Alarm Color"=w1089, "Alarm Status"=w1088) -> (w1094:T7)
            }
          }
          n533 = Replace Array Subset(array=w1049, new element=w1061, index (row)=w1048, index (col)=w1047) -> (w1042:T3)
        }
        n534 = local write "Thermocouples"(w1011) -> ()
        n535 = Bundle By Name(cluster=w1018, "Thermocouples"=w1011, "working array"=w1017) -> (w1012:T6)
        n536 = Build Array (concatenate)(waveform(dbl) {"t0"=timestamp(0 s since 1904-01-01), "dt"=1.0, "Y"=[]} ("element"), w1009) -> (w1021:waveform(dbl)[])
        n537 = Delete From Array(array=w1021, index=0) -> (array with subset deleted=→"Waveform Chart":waveform(dbl)[])  [unwired: 1 in, 1 out]
      }
      frame "getTemps" {
        n538 = Unbundle By Name(w1121) -> ("Http session"=w1125:T5, "URL prefex"=w1123:string, "PumpTemps"=w1116:T4)
        n539 = local read "Local Debug"() -> (w1118:bool)
        n540 = Concatenate Strings(w1123, "getMCCData" ("url")) -> (w1124:string)
        n541 = case shown="False" w1118 {
          tunnel: w1125 -> [w1130 w1165]
          tunnel: w1124 -> [w1131 w1164]
          tunnel: w1120 -> [_ w1162]
          tunnel: [w1128 w1161] -> w1119
          tunnel: "Read MCC" -> [w1129 _]
          tunnel: w1116 -> [w1127 w1149]
          frame False {
            n542 = case shown="False" w1129 {
              tunnel: w1131 -> [_ w1136]
              tunnel: w1130 -> [_ w1135]
              tunnel: [w1132 w1134] -> w1128
              tunnel: w1127 -> [w1132 w1133]
              frame False {
              }
              frame True {
                n543 = call <vilib>:"GET.vi"("client handle"=w1135, "url"=w1136) -> ("body"=w1137:string)  [unwired: 10 in, 3 out]
                n544 = Unflatten From JSON(JSON string=w1137, type and defaults=T9 {"DutyCycle"=0, "Stage1Temp"=0, "CryoPumpReadyState"={"MotorOn"=FALSE, "Ready"=FALSE}, "PurgeValveState"=FALSE, "RegenError"="", "RegenStep"="", "RoughingValveState"=FALSE, "RoughingInterlock"={"RoughingPermission"=FALSE, "RoughingNeeded"=FALSE, "Cryopumprunning"=FALSE}, "Stage2Temp"=0, "Status"={"PumpOn"=FALSE, "RoughOpen"=FALSE, "PurgeOpen"=FALSE, "ThermocoupleGaugeOn"=FALSE, "PowerFailureOccurred"=FALSE}, "TcPressure"=0}) -> (value=w1148:T9)  [unwired: 5 in, 1 out]
                n545 = Unbundle By Name(w1148) -> ("Stage1Temp"=w1146:i32, "Stage2Temp"=w1145:i32, "TcPressure"=w1144:i32)
                n546 = To Double Precision Float(number=w1146) -> (double precision float=w1143:dbl)
                n547 = To Double Precision Float(number=w1145) -> (double precision float=w1142:dbl)
                n548 = To Double Precision Float(number=w1144) -> (double precision float=w1141:dbl)
                n549 = Build Array(w1142) -> (w1139:dbl[])
                n550 = Build Array(w1141) -> (w1140:dbl[])
                n551 = Build Array(w1143) -> (w1138:dbl[])
                n552 = Bundle(cluster=w1133, "Cp Stage 1 Temp"=w1138, "Cp Stage 2 Temp"=w1139, "Compressor Temp"=w1140) -> (w1134:T4)
              }
            }
          }
          frame True {
            n553 = call-poly <vilib>:"POST.vi"("client handle"=w1165, "url"=w1164, "error in (no error)"=w1162) -> ("body"=w1163:string)  [unwired: 9 in, 3 out]
            n554 = Unflatten From JSON(JSON string=w1163, type and defaults=T9 {"DutyCycle"=0, "Stage1Temp"=0, "CryoPumpReadyState"={"MotorOn"=FALSE, "Ready"=FALSE}, "PurgeValveState"=FALSE, "RegenError"="", "RegenStep"="", "RoughingValveState"=FALSE, "RoughingInterlock"={"RoughingPermission"=FALSE, "RoughingNeeded"=FALSE, "Cryopumprunning"=FALSE}, "Stage2Temp"=0, "Status"={"PumpOn"=FALSE, "RoughOpen"=FALSE, "PurgeOpen"=FALSE, "ThermocoupleGaugeOn"=FALSE, "PowerFailureOccurred"=FALSE}, "TcPressure"=0}) -> (value=w1160:T9)  [unwired: 5 in, 1 out]
            n555 = Unbundle By Name(w1160) -> ("Stage1Temp"=w1158:i32, "Stage2Temp"=w1157:i32, "TcPressure"=w1156:i32)
            n556 = To Double Precision Float(number=w1158) -> (double precision float=w1155:dbl)
            n557 = To Double Precision Float(number=w1157) -> (double precision float=w1154:dbl)
            n558 = To Double Precision Float(number=w1156) -> (double precision float=w1153:dbl)
            n559 = Build Array(w1154) -> (w1151:dbl[])
            n560 = Build Array(w1153) -> (w1152:dbl[])
            n561 = Build Array(w1155) -> (w1150:dbl[])
            n562 = Bundle(cluster=w1149, "Cp Stage 1 Temp"=w1150, "Cp Stage 2 Temp"=w1151, "Compressor Temp"=w1152) -> (w1161:T4)
          }
        }
        n563 = Bundle By Name(cluster=w1121, "PumpTemps"=w1119) -> (w1126:T6)
      }
      frame "getThermalProfile" {
        n564 = Unbundle By Name(w1169) -> ("Http session"=w1173:T5, "URL prefex"=w1171:string)
        n565 = local read "Local Debug"() -> (w1168:bool)
        n566 = case shown="True" "ThermalProfile" {
          tunnel: w1173 -> [_ w1183]
          tunnel: "getAllZoneData" ("url") -> [_ w1181]
          tunnel: w1171 -> [_ w1178]
          tunnel: cluster{"ZoneSetPoint":dbl[], "ZoneTemp":dbl[]} {"ZoneSetPoint"=[], "ZoneTemp"=[]} -> [_ w1177]
          tunnel: w1168 -> [_ w1176]
          frame False {
          }
          frame True {
            n567 = Flatten To JSON(anything=w1177) -> (JSON string=w1180:string)  [unwired: 2 in, 1 out]
            n568 = Concatenate Strings(w1178, w1181) -> (w1182:string)
            n569 = case shown="True" w1176 {
              tunnel: [w1188 w1189] -> _
              tunnel: [w1187 w1190] -> _
              tunnel: w1183 -> [_ _]
              tunnel: w1182 -> [w1186 w1193]
              tunnel: [w1185 w1191] -> w1179
              tunnel: [w1184 w1192] -> w1174
              tunnel: w1180 -> [_ w1194]
              frame False {
                n570 = call <vilib>:"GET.vi"("url"=w1186) -> ("client handle out"=w1187:T5, "headers"=w1184:string, "body"=w1185:string, "error out"=w1188:errorcluster)  [unwired: 11 in]
              }
              frame True {
                n571 = call-poly <vilib>:"POST.vi"("url"=w1193, "buffer"=w1194) -> ("client handle out"=w1190:T5, "headers"=w1192:string, "body"=w1191:string, "error out"=w1189:errorcluster)  [unwired: 10 in]
              }
            }
            "headers" <- w1174
            n572 = Unflatten From JSON(JSON string=w1179, type and defaults=w1177) -> (value=→"value":cluster{"ZoneSetPoint":dbl[], "ZoneTemp":dbl[]})  [unwired: 5 in, 1 out]
          }
        }
      }
      frame "getZones" {
        n573 = Unbundle By Name(w1205) -> ("Http session"=w1208:T5, "URL prefex"=w1203:string)
        n574 = Concatenate Strings(w1203, "getZoneTemps" ("url")) -> (w1207:string)
        n575 = local read "Local Debug"() -> (w1204:bool)
        n576 = case shown="True" "Read Zones" {
          tunnel: w1208 -> [_ w1219]
          tunnel: w1207 -> [_ w1218]
          tunnel: w1204 -> [_ w1215]
          tunnel: [_ w1212] -> w1199
          tunnel: [_ w1211] -> w1197
          frame False {
          }
          frame True {
            w1214 = cluster{"ZoneSetPoint":dbl[], "ZoneTemp":dbl[]} {"ZoneSetPoint"=[], "ZoneTemp"=[]}
            n577 = Flatten To JSON(anything=w1214) -> (JSON string=w1217:string)  [unwired: 2 in, 1 out]
            n578 = case shown="True" w1215 {
              tunnel: [w1224 w1225] -> _
              tunnel: [w1223 w1226] -> _
              tunnel: w1219 -> [_ _]
              tunnel: w1218 -> [w1222 w1229]
              tunnel: [w1221 w1227] -> w1216
              tunnel: [w1220 w1228] -> _
              tunnel: w1217 -> [_ w1230]
              frame False {
                n579 = call <vilib>:"GET.vi"("url"=w1222) -> ("client handle out"=w1223:T5, "headers"=w1220:string, "body"=w1221:string, "error out"=w1224:errorcluster)  [unwired: 11 in]
              }
              frame True {
                n580 = call-poly <vilib>:"POST.vi"("url"=w1229, "buffer"=w1230) -> ("client handle out"=w1226:T5, "headers"=w1228:string, "body"=w1227:string, "error out"=w1225:errorcluster)  [unwired: 10 in]
              }
            }
            n581 = Unflatten From JSON(JSON string=w1216, type and defaults=w1214) -> (value=w1213:cluster{"ZoneSetPoint":dbl[], "ZoneTemp":dbl[]})  [unwired: 5 in, 1 out]
            n582 = Unbundle By Name(w1213) -> ("ZoneSetPoint"=w1211:dbl[], "ZoneTemp"=w1212:dbl[])
          }
        }
        n583 = Initialize Array(0.0 ("element"), 18 ("dimension size")) -> (w1200:dbl[])
        n584 = for {
          N: 18 -> [_]
          tunnel: w1199 -> [w1232]
          shift-right: [w1231] -> w1196
          shift-left: w1200 -> [w1236]
          tunnel: w1197 -> [w1233]
          i -> [w1235]
          n585 = Quotient & Remainder(x=w1235, y=2) -> (x-y*floor(x/y)=w1234:i32)  [unwired: 1 out]
          n586 = Equal To 0?(x=w1234) -> (x = 0?=w1237:bool)
          n587 = case shown="False" w1237 {
            tunnel: w1236 -> [w1245 w1252]
            tunnel: w1235 -> [w1240 w1249]
            tunnel: [w1244 w1251] -> w1231
            tunnel: w1233 -> [w1241 _]
            tunnel: w1232 -> [_ w1250]
            frame False {
              n588 = Quotient & Remainder(x=w1240, y=2) -> (floor(x/y)=w1242:i32)  [unwired: 1 out]
              n589 = Index Array(array=w1241, index=w1242) -> (element=w1239:dbl)
              n590 = Replace Array Subset(array=w1245, new element=w1239, index=w1240) -> (w1244:dbl[])
            }
            frame True {
              n591 = Quotient & Remainder(x=w1249, y=2) -> (floor(x/y)=w1247:i32)  [unwired: 1 out]
              n592 = Index Array(array=w1250, index=w1247) -> (element=w1246:dbl)
              n593 = Replace Array Subset(array=w1252, new element=w1246, index=w1249) -> (w1251:dbl[])
            }
          }
        }
        n594 = Bundle By Name(cluster=w1205, "Zones"=w1196) -> (w1209:T6)
      }
      frame "masterDatabase" {
        n595 = Unbundle By Name(w1264) -> ("Thermocouples"=w1265:T3, "Pressure"=w1256:dbl[], "PumpTemps"=w1260:T4, "NumberTCs"=w1266:i32, "Zones"=w1253:dbl[])  [unwired: 1 out]
        n596 = Initialize Array(0.0 ("element"), w1266) -> (w1268:dbl[])
        n597 = Unbundle(w1260) -> ("Cp Stage 1 Temp"=w1259:dbl[], "Cp Stage 2 Temp"=w1258:dbl[], "Compressor Temp"=w1257:dbl[])
        n598 = Build Array (concatenate)(w1259, w1258, w1257) -> (w1255:dbl[])
        n599 = for {
          N: w1266 -> [_]
          shift-right: [w1278] -> w1254
          shift-left: w1268 -> [w1279]
          tunnel: w1265 -> [w1274]
          i -> [w1276]
          n600 = Quotient & Remainder(x=w1276, y=4) -> (x-y*floor(x/y)=w1273:i32, floor(x/y)=w1275:i32)
          n601 = Index Array(array=w1274, index (row)=w1275, index (col)=w1273) -> (element=w1272:T7)
          n602 = Unbundle By Name(w1272) -> ("Temperature"=w1271:string)
          n603 = Fract/Exp String To Number(string=w1271) -> (number=w1270:dbl)  [unwired: 3 in, 1 out]
          n604 = To Double Precision Float(number=w1270) -> (double precision float=w1280:dbl)
          n605 = Replace Array Subset(array=w1279, new element=w1280, index=w1276) -> (w1278:dbl[])
        }
        n606 = Build Array (concatenate)(dbl[] [0.0], w1256, w1253, w1254, w1255) -> (w1262:dbl[])
        n607 = Bundle By Name(cluster=w1264, "Database"=w1262) -> (w1263:T6)
      }
      frame "multipleGraphs" {
        n608 = local read "Custom Graph Selector"() -> (w1281:i32)
        n609 = for {
          N: 6 ("Numeric") -> [_]
          tunnel: w1284 -> [w1298]
          tunnel: w1283 -> [w1297]
          tunnel: w1281 -> [w1288]
          i -> [w1285]
          n610 = case shown="2" w1285 {
            tunnel: [w1344 w1345 w1347 w1349 w1351 w1353] -> w1290
            tunnel: [w1343 w1346 w1348 w1350 w1352 w1354] -> w1289
            frame 0, Default {
              n611 = control-ref of="Custom Chart 1 Selection"() -> (w1343:refnum<vi>)
              n612 = control-ref of="Custom Chart 1"() -> (w1344:refnum<vi>)
            }
            frame 1 {
              n613 = control-ref of="Custom Chart 2 Selection"() -> (w1346:refnum<vi>)
              n614 = control-ref of="Custom Chart 2"() -> (w1345:refnum<vi>)
            }
            frame 2 {
              n615 = control-ref of="Custom Chart 3 Selection"() -> (w1348:refnum<vi>)
              n616 = control-ref of="Custom Chart 3"() -> (w1347:refnum<vi>)
            }
            frame 3 {
              n617 = control-ref of="Custom Chart 4 Selection"() -> (w1350:refnum<vi>)
              n618 = control-ref of="Custom Chart 4"() -> (w1349:refnum<vi>)
            }
            frame 4 {
              n619 = control-ref of="Custom Chart 5 Selection"() -> (w1352:refnum<vi>)
              n620 = control-ref of="Custom Chart 5"() -> (w1351:refnum<vi>)
            }
            frame 5 {
              n621 = control-ref of="Custom Chart 6 Selection"() -> (w1354:refnum<vi>)
              n622 = control-ref of="Custom Chart 6"() -> (w1353:refnum<vi>)
            }
          }
          n623 = Equal?(x=w1288, y=w1285) -> (x = y?=w1286:bool)
          n624 = Unbundle By Name(w1297) -> ("Database"=w1295:dbl[], "numSensors"=w1296:i32)
          n625 = case shown="True" w1286 {
            tunnel: w1298 -> [_ w1312]
            tunnel: [w1301 w1306] -> w1294
            tunnel: [1000 w1305] -> w1293
            tunnel: w1289 -> [w1302 w1304]
            tunnel: [FALSE w1303] -> w1287
            frame False {
              n626 = property on="Property Node" class="LstBox (strict)"(reference=w1302) -> ("Item Symbols"=w1301:i32[])  [unwired: 1 in, 2 out]
            }
            frame True {
              n627 = property on="Property Node" class="LstBox (strict)"(reference=w1304) -> ("Item Symbols"=w1306:i32[])  [unwired: 1 in, 2 out]
              n628 = Decimal String To Number(string=w1312) -> (number=w1305:i32)  [unwired: 2 in, 1 out]
              n629 = Index Array(array=w1306, index=0) -> (element=w1307:i32)
              n630 = Equal?(x=37, y=w1307) -> (x = y?=w1309:bool)
              n631 = Equal To 0?(x=w1305) -> (x = 0?=w1311:bool)
              n632 = And(x=w1309, y=w1311) -> (x .and. y?=w1303:bool)
            }
          }
          n633 = case shown="True" w1287 {
            tunnel: [0 ("index") w1407] -> w1292
            tunnel: w1296 -> [w1361 w1403]
            tunnel: w1295 -> [w1360 _]
            tunnel: [w1359 _] -> w1291
            tunnel: w1293 -> [w1357 w1407]
            tunnel: w1294 -> [w1358 w1406]
            tunnel: w1289 -> [w1356 w1402]
            tunnel: w1290 -> [w1355 w1401]
            frame False {
              n634 = for {
                N: w1361 -> [_]
                tunnel: [w1380] -> w1359 mode=indexing
                tunnel: w1357 -> [w1374]
                tunnel: w1358 -> [w1369]
                tunnel: w1360 -> [w1366] mode=indexing
                tunnel: w1356 -> [w1364]
                tunnel: w1355 -> [w1363]
                i -> [w1367]
                n635 = Wait (ms)(milliseconds to wait=u32 0) -> ()  [unwired: 1 out]
                n636 = Get Date/Time In Seconds() -> (seconds since 1Jan1904=w1382:timestamp)
                n637 = Bundle By Name("t0"=w1382) -> (w1381:waveform(dbl))  [unwired: 1 in]
                n638 = Build Array(w1366) -> (w1365:dbl[])
                n639 = Bundle By Name(cluster=w1381, "Y"=w1365) -> (w1380:waveform(dbl))
                n640 = Index Array(array=w1369, index=w1374) -> (element=w1372:i32)
                n641 = Index Array(array=w1369, index=w1374) -> (element=w1375:i32)
                n642 = Equal?(x=w1372, y=38) -> (x = y?=w1371:bool)
                n643 = Equal?(x=w1375, y=37) -> (x = y?=w1377:bool)
                n644 = Equal?(x=w1367, y=w1374) -> (x = y?=w1370:bool)
                n645 = And(x=w1370, y=w1371) -> (x .and. y?=w1368:bool)
                n646 = And(x=w1370, y=w1377) -> (x .and. y?=w1376:bool)
                n647 = case shown="True" w1376 {
                  tunnel: w1369 -> [_ w1400]
                  tunnel: w1374 -> [_ _]
                  tunnel: w1367 -> [_ w1395]
                  tunnel: w1363 -> [_ w1392]
                  tunnel: w1364 -> [_ w1393]
                  frame False {
                  }
                  frame True {
                    n648 = property on="Property Node" class="WFChart (strict)"(reference=w1392, "Active Plot"=w1395) -> (reference out=w1398:refnum<vi>)  [unwired: 1 in, 1 out]
                    n649 = Replace Array Subset(array=w1400, new element=38, index=w1395) -> (w1396:i32[])
                    n650 = property on="Property Node" class="WFChart (strict)"(reference=w1392) -> ("Plot.Plot Color"=w1394:u32)  [unwired: 1 in, 2 out]
                    n651 = property on="Property Node" class="WFChart (strict)"(reference=w1398, "Plot.Visible?"=TRUE ("Plot.Visible")) -> ()  [unwired: 1 in, 2 out]
                    n652 = property on="Property Node" class="LstBox (strict)"(reference=w1393, "Active Row"=w1395) -> ()  [unwired: 1 in, 2 out]
                    n653 = property on="Property Node" class="LstBox (strict)"(reference=w1393, "CellBG"=w1394) -> ()  [unwired: 1 in, 2 out]
                    n654 = property on="Property Node" class="LstBox (strict)"(reference=w1393, "Item Symbols"=w1396) -> ()  [unwired: 1 in, 2 out]
                  }
                }
                n655 = case shown="True" w1368 {
                  tunnel: w1369 -> [_ w1391]
                  tunnel: w1367 -> [_ w1384]
                  tunnel: w1363 -> [_ w1385]
                  tunnel: w1364 -> [_ w1386]
                  frame False {
                  }
                  frame True {
                    n656 = property on="Property Node" class="WFChart (strict)"(reference=w1385, "Active Plot"=w1384) -> (reference out=w1389:refnum<vi>)  [unwired: 1 in, 1 out]
                    n657 = Replace Array Subset(array=w1391, new element=37, index=w1384) -> (w1387:i32[])
                    n658 = property on="Property Node" class="WFChart (strict)"(reference=w1389, "Plot.Visible?"=FALSE ("Plot.Visible")) -> ()  [unwired: 1 in, 2 out]
                    n659 = property on="Property Node" class="LstBox (strict)"(reference=w1386, "Active Row"=w1384) -> ()  [unwired: 1 in, 2 out]
                    n660 = property on="Property Node" class="LstBox (strict)"(reference=w1386, "CellBG"=u32 13816530 ("Active Row:Cell Background Color")) -> ()  [unwired: 1 in, 2 out]
                    n661 = property on="Property Node" class="LstBox (strict)"(reference=w1386, "Item Symbols"=w1387) -> ()  [unwired: 1 in, 2 out]
                  }
                }
              }
            }
            frame True {
              n662 = for {
                N: w1403 -> [_]
                tunnel: w1406 -> [_]
                tunnel: w1402 -> [w1409]
                tunnel: w1401 -> [w1408]
                i -> [w1410]
                n663 = property on="Property Node" class="WFChart (strict)"(reference=w1408, "Active Plot"=w1410) -> (reference out=w1413:refnum<vi>)  [unwired: 1 in, 1 out]
                n664 = property on="Property Node" class="WFChart (strict)"(reference=w1413, "Plot.Visible?"=FALSE ("Plot.Visible")) -> ()  [unwired: 1 in, 2 out]
                n665 = property on="Property Node" class="LstBox (strict)"(reference=w1409, "Active Row"=w1410) -> ()  [unwired: 1 in, 2 out]
                n666 = property on="Property Node" class="LstBox (strict)"(reference=w1409, "CellBG"=u32 13816530 ("Active Row:Cell Background Color")) -> ()  [unwired: 1 in, 2 out]
              }
              n667 = Initialize Array(37, w1403) -> (w1404:i32[])
              n668 = property on="Property Node" class="LstBox (strict)"(reference=w1402, "Item Symbols"=w1404) -> ()  [unwired: 1 in, 2 out]
            }
          }
          n669 = case shown="5" w1285 {
            tunnel: w1292 -> [w1314 w1319 w1324 w1329 w1334 w1339]
            tunnel: w1291 -> [w1313 w1318 w1323 w1328 w1333 w1338]
            frame 0, Default {
              n670 = Build Array (concatenate)(waveform(dbl) {"t0"=timestamp(0 s since 1904-01-01), "dt"=1.0, "Y"=[]} ("element"), w1313) -> (w1317:waveform(dbl)[])
              n671 = Delete From Array(array=w1317, index=w1314) -> (array with subset deleted=→"Custom Chart 1":waveform(dbl)[])  [unwired: 1 in, 1 out]
            }
            frame 1 {
              n672 = Build Array (concatenate)(waveform(dbl) {"t0"=timestamp(0 s since 1904-01-01), "dt"=1.0, "Y"=[]} ("element"), w1318) -> (w1322:waveform(dbl)[])
              n673 = Delete From Array(array=w1322, index=w1319) -> (array with subset deleted=→"Custom Chart 2":waveform(dbl)[])  [unwired: 1 in, 1 out]
            }
            frame 2 {
              n674 = Build Array (concatenate)(waveform(dbl) {"t0"=timestamp(0 s since 1904-01-01), "dt"=1.0, "Y"=[]} ("element"), w1323) -> (w1327:waveform(dbl)[])
              n675 = Delete From Array(array=w1327, index=w1324) -> (array with subset deleted=→"Custom Chart 3":waveform(dbl)[])  [unwired: 1 in, 1 out]
            }
            frame 3 {
              n676 = Build Array (concatenate)(waveform(dbl) {"t0"=timestamp(0 s since 1904-01-01), "dt"=1.0, "Y"=[]} ("element"), w1328) -> (w1332:waveform(dbl)[])
              n677 = Delete From Array(array=w1332, index=w1329) -> (array with subset deleted=→"Custom Chart 4":waveform(dbl)[])  [unwired: 1 in, 1 out]
            }
            frame 4 {
              n678 = Build Array (concatenate)(waveform(dbl) {"t0"=timestamp(0 s since 1904-01-01), "dt"=1.0, "Y"=[]} ("element"), w1333) -> (w1337:waveform(dbl)[])
              n679 = Delete From Array(array=w1337, index=w1334) -> (array with subset deleted=→"Custom Chart 5":waveform(dbl)[])  [unwired: 1 in, 1 out]
            }
            frame 5 {
              n680 = Build Array (concatenate)(waveform(dbl) {"t0"=timestamp(0 s since 1904-01-01), "dt"=1.0, "Y"=[]} ("element"), w1338) -> (w1342:waveform(dbl)[])
              n681 = Delete From Array(array=w1342, index=w1339) -> (array with subset deleted=→"Custom Chart 6":waveform(dbl)[])  [unwired: 1 in, 1 out]
            }
          }
        }
      }
      frame "setThermalProfile" {
        n682 = event shown="[0] \"Set Z 1\": Mouse Down" {
          selector: _ -> [_]
          dyn-events: _ -> [_]
          timeout: _ -> [_]
          tunnel: T2 {"profiles"=[]} -> [w1423]
          event "Set Z 1": Mouse Down {
            n683 = event-data() -> ()  [unwired: 1 in, 8 out]
            n684 = local read "Cluster"() -> (w1417:T2)
            n685 = Unbundle By Name(w1417) -> ("profiles"=w1418:T15)
            n686 = Array To Cluster(array=w1418) -> (cluster=w1422:T16)
            n687 = local read "Zone 1 Temp"() -> (w1420:u16)
            n688 = Unbundle By Name(w1422) -> ("profiles[0]"=w1421:T1)
            n689 = Bundle By Name(cluster=w1421, "zone"=1, "average"=w1420) -> (→"output cluster":T1)
            "Cluster" <- w1423
          }
        }
      }
      frame "exit" {
        n690 = Unbundle By Name(w1425) -> ("Http session"=w1426:T5)
        n691 = call <vilib>:"CloseHandle.vi"("client handle"=w1426, "error in (no error)"=w1428) -> ("error out"=w1427:errorcluster)  [unwired: 13 in]
        n692 = Bundle By Name(cluster=w1425, "go"=FALSE ("Bundle Element")) -> (w1429:T6)
      }
      frame Default {
        n693 = call "Unknown Message Dialog.vi"("error in (no error)"=w1432, "event name"=w1431) -> ("error out"=w1430:errorcluster)  [unwired: 9 in]
      }
    }
    n694 = Unbundle By Name(w30) -> ("go"=w29:bool)
    n695 = call "log system event.vi"("error in (no error)"=w32) -> ("error out"=w31:errorcluster)  [unwired: 9 in, 1 out]
  }
  n696 = call "Unload Module.vi"("error in (no error)"=w9) -> ()  [unwired: 10 in, 1 out]
  n697 = property on="Waveform Chart" class="WFChart (strict)" props=["Plot", "Visible?"]() -> ()  [unwired: 2 in, 3 out]
